vi "POM_PROM_ТЗЧ_host.vi"() -> ()   [LabVIEW 2013]
uses:
  <instrlib>/niDMM/nidmm.llb/niDMM Resolution in Digits.ctl
  <instrlib>/niDMM/nidmm.llb/niDMM Function.ctl
  <vilib>/Analysis/baseanly.llb/Mean (DBL).vi
  <instrlib>/niDMM/nidmm.llb/niDMM Configure Measurement Digits.vi
  <vilib>/Analysis/NI_AALBase.lvlib
  <instrlib>/niDCPower/nidcpower.llb/niDCPower Measurement Type.ctl
panel:
  in  "Нагрев":bool
  in  "В ручную":bool
  in  "Напряжение Пельтье":dbl=0.30000000000000004
  in  "milliseconds to wait 2":u32=75
  out "Monitor current, uA":dbl(graph)=0.07016814151938888
  in  "Порог типатиристора, мА":dbl=55.0
  out "Счетчик сбоев":dbl
  out "Температура":i32=25
  out "Образец":i32=2001
  out "Сеанс":i32
  out "Ион":string="Nope"
  in  "SEL simulation":bool
  out "refnum out":refnum<file>
  in  "Облучение!":bool
  out "Стабилизировано":bool
  in  "+ V TEC для новой точки":dbl=0.11 format="%#_13g"
  in  "Вычет для \"антиразгона\"":dbl format="%#_13g"
  in  "Оставить в раб.\nрежиме":bool
  out "Boolean":bool
  in  "Num_hits_req":u64=7
  out "Num_hits":u64
  in  "Count_hits?":bool
  in  "tstab между точками, мс":u32=1
  in  "Предел тока PDext, мА":dbl=20.0
  in  "Отладка(F)/\n/Рабочий(T)":bool=TRUE
  out "TEC_current, mA":dbl=27.478324133936702
  in  "Param_Log":path=path "D:/#rkm/FONONIWE-4/Logs_Dubna/POM"
  in  "trelax":u32=35000
  out "Volt_onRes":dbl=2.4602762193630356
  out "NoStab":bool
  out "Operating Current, mA":dbl=0.04490127125944435
  in  "Desirable Operating current, mA":dbl=50.0 format="%#_6f"
  out "Error message":string="Too much try"
  in  "Up_Volt_limit":dbl=5.0
  in  "Low_Volt_limit":dbl=1.0
  out "ThRes_stabil":bool=TRUE
  out "Подстроенное напряжение\nстабилизации":dbl=0.15911789062499992
  out "ThRes value":dbl=17926.2140625
  in  "Optimum ThRes":dbl=18000.0 format="%#_6f"
  in  "Предел тока LD, мА":dbl=100.0
  in  "Предел тока ТЕС, мА":dbl=300.0
  in  "Tab Control":enum32{"Page 1", "Page 2", "Page 3", "Page 4"}(tab)=enum."Page 4"
  out "RES(U_TEC) Graph":cluster{dbl[], dbl[]}(graph)={[-0.0, 0.025, 0.05, 0.07500000000000001, 0.1, 0.125, 0.15, 0.175, 0.19999999999999998, 0.22499999999999998, 0.24999999999999997, 0.27499999999999997, 0.3, 0.325, 0.35000000000000003, 0.37500000000000006, 0.4000000000000001, 0.4250000000000001, 0.4500000000000001, 0.47500000000000014, 0.5000000000000001, 0.5250000000000001, 0.5500000000000002, 0.5750000000000002, 0.6000000000000002, 0.6250000000000002, 0.6500000000000002, 0.6750000000000003, 0.7000000000000003, 0.7250000000000003, 0.7500000000000003, 0.7750000000000004], [15319.04365234375, 15328.19267578125, 15358.49169921875, 15409.562109375, 15479.3826171875, 15563.1861328125, 15668.50888671875, 15780.12734375, 15906.40224609375, 16043.244921875, 16186.97255859375, 16341.84609375, 16507.0697265625, 16676.522265625, 16856.963671875, 17044.884375, 17239.0294921875, 17436.3736328125, 17641.744140625, 17850.8728515625, 18071.7896484375, 18291.20625, 18518.965625, 18750.4271484375, 18987.4517578125, 19230.0744140625, 19480.026171875, 19731.8517578125, 19984.940234375, 20249.54140625, 20514.206640625, 20780.055078125]}
  out "RES(I_TEC) Graph":cluster{dbl[], dbl[]}(graph)={[0.03457500435386299, 4.049114950716204, 7.9212407853678135, 11.611043015146826, 15.078954849250364, 18.53827902856892, 21.88408259580828, 25.295266856430793, 28.546483256934756, 31.60504570629327, 34.77027313644012, 37.80993408960394, 40.856486299311584, 43.94949565069024, 47.03219408159836, 50.06845592920464, 52.92926046093485, 55.95350027659507, 58.865931959242474, 61.84202368829837, 64.7802788203752, 67.60156326899994, 70.44177990185035, 73.41963022613506, 76.46974363403558, 79.22741287887104, 82.2001312992484, 85.07135997639818, 88.0785044464861, 90.98931976346292, 93.95691599392462, 96.75420696595256], [15319.04365234375, 15328.19267578125, 15358.49169921875, 15409.562109375, 15479.3826171875, 15563.1861328125, 15668.50888671875, 15780.12734375, 15906.40224609375, 16043.244921875, 16186.97255859375, 16341.84609375, 16507.0697265625, 16676.522265625, 16856.963671875, 17044.884375, 17239.0294921875, 17436.3736328125, 17641.744140625, 17850.8728515625, 18071.7896484375, 18291.20625, 18518.965625, 18750.4271484375, 18987.4517578125, 19230.0744140625, 19480.026171875, 19731.8517578125, 19984.940234375, 20249.54140625, 20514.206640625, 20780.055078125]}
  out "I_PD_Ext(I_LD) Graph":cluster{dbl[], dbl[]}(graph)={[0.0, 5.125820672560687, 10.202363077068034, 15.09070291650038, 20.026524721844005, 24.848748653112324, 29.706585438813228, 34.55255888002156, 39.41379829521783, 44.31743313126964, 49.35841653002704], [0.6213749657825949, 0.6126206411732633, 0.5986137214569519, 0.5846068013204628, 0.5933611264550083, 0.5670981505590477, 0.5355825775341941, 0.586357666360488, 0.5355825775341941, 0.5478386339632713, 0.5390843079753067]}
  out "I_PD(I_LD) Graph":cluster{dbl[], dbl[]}(graph)={[0.0, 5.125820672560687, 10.202363077068034, 15.09070291650038, 20.026524721844005, 24.848748653112324, 29.706585438813228, 34.55255888002156, 39.41379829521783, 44.31743313126964, 49.35841653002704], [0.00446055423708458, 0.1890051237296575, 1.3185992656872259, 47.69851657329127, 96.3842059718445, 145.3466946259141, 195.95923949964345, 243.1108383461833, 288.08951028622687, 334.6654470078647, 377.8655605856329]}
  out "I_pd, uA":dbl
  out "IPD(ext), mA":dbl
  out "V2(I_LD) Graph":cluster{dbl[], dbl[]}(graph)={[0.0, 5.125820672560687, 10.202363077068034, 15.09070291650038, 20.026524721844005, 24.848748653112324, 29.706585438813228, 34.55255888002156, 39.41379829521783, 44.31743313126964, 49.35841653002704], [0.0006418486043783589, 1.1699665507043246, 1.452329111789965, 1.6798119558569469, 1.9201177244634586, 2.150803801269446, 2.3862573437846697, 2.612869753183121, 2.8439823589319366, 3.0683008415602466, 3.3013683877429134]}
  out "Forward Voltage, V":dbl
  out "OP(I_LD) Graph":cluster{dbl[], dbl[]}(graph)={[0.0, 5.125820672560687, 10.202363077068034, 15.09070291650038, 20.026524721844005, 24.848748653112324, 29.706585438813228, 34.55255888002156, 39.41379829521783, 44.31743313126964, 49.35841653002704], [0.0, 0.0, 0.02, 0.74, 1.5, 2.27, 3.0300000000000002, 3.8, 4.58, 5.33, 6.119999999999999]}
  out "Ophir, mW":dbl
  out "Пороговый ток":dbl
  out "ExtPhotodiode Current":dbl(graph)
  out "Boolean 2":bool
  out "Сопротивление терморез-ра":dbl(graph)=16035.80078125
  out "thRes_adj":dbl=16035.80078125 format="%0.2f"
  in  "Source-Ohm w8":u32=1000
  in  "Coeff_High":dbl=90000.0 format="%#_13g"
  in  "Coeff_low":dbl=20000.0 format="%#_13g"
  in  "Coeff_thr":dbl=1500.0
  out "+Voltage\nrequired":dbl=0.0008410915798611111
  out "Разница ThRes":dbl=75.6982421875
  out "Operating Current":dbl(graph)
  out "Готовы облучать":bool
  out "accommodated voltage (out)":dbl=5.701287315779691
  in  "4070_Rele_source":enum16{"S2_Ch0", "S1_Ch2"}(ring)
  in  "the upper limit for the voltage_LD":dbl=6.0
  in  "the lower limit for the voltage_LD":dbl=1.0
  in  "Start voltage_LD":dbl=2.0 format="%#.7f"
  in  "accuracy_LD":dbl=0.01 step=0.01
  in  "Res_LD":dbl=50.0
  in  "TEC_Source":enum16{"S1_Ch2", "S2_Ch0", "S3_Ch1"}(ring)
  in  "Start voltage":dbl=0.1 format="%#.7f"
  in  "the upper limit for the voltage":dbl=0.8
  in  "the lower limit for the voltage":dbl
  in  "Точность ThRes":dbl=75.0 step=0.01
  out "Ro, Ом":dbl=15321.56484375
  in  "OphirLMMeasurementLib.ICoLMMeasurement":refnum<k7>
  out "hDevice":i32=1004
  out "Ophir_address":refnum<k7>
  in  "Power Enable":bool
  in  "4071(2)":refnum<k15>="PXI1Slot4_2"
  out "4071(2)_adress":refnum<k15>="PXI1Slot4_2 (12)" caption="4071(1)_out"
  in  "4071(1)":refnum<k15>="Dev5"
  out "4071(1)_adress":refnum<k15>="Dev5 (5)" caption="4071(1)_out"
  out "4070_address":refnum<k15>="PXI4Slot10 (5)" caption="4070_out"
  in  "4070":refnum<k15>="PXI4Slot10"
  in  "Source_3":refnum<k15>
  out "Source_3_Vcc_out":refnum<k15> caption="S_3_out"
  out "Source_2_Vcc_out":refnum<k15>="PXI4Slot2" caption="S_2_out"
  in  "Source_2":refnum<k15>="PXI4Slot2"
  out "Source_1_Vcc_out":refnum<k15>="PXI4Slot4" caption="S_1_out"
  in  "Source_1":refnum<k15>="PXI4Slot4"
  out "Прервать":bool=TRUE
  in  "milliseconds to wait":u32=2000
  in  "Шаг напр\nдля TEC, В":dbl=0.025
  in  "Начальное\nнапряжение TEC, В":dbl
  in  "кол-во точек для TEC":i32=32
  in  "stop":bool
  in  "Case":T1(ring)=enum."Quit"
  out "Выполняется":bool
  in  "Раб. режим LD":bool
  in  "Хар-ка TEC":bool
  in  "Хар-ки от I_LD":bool
  out "Status:":string="IDLE"
  out "Подстроенный ток, mA":dbl=50.042267338193476
  in  "Шаг, мА":dbl=5.0
  in  "Начальный ток, мА":dbl
  in  "Кол-во точек":i32=11
  # "20"
  # "7"
  # "5"
  # "ток Пельтье во время стабилизации"
  # "0,15"
  # "Охлаждение"
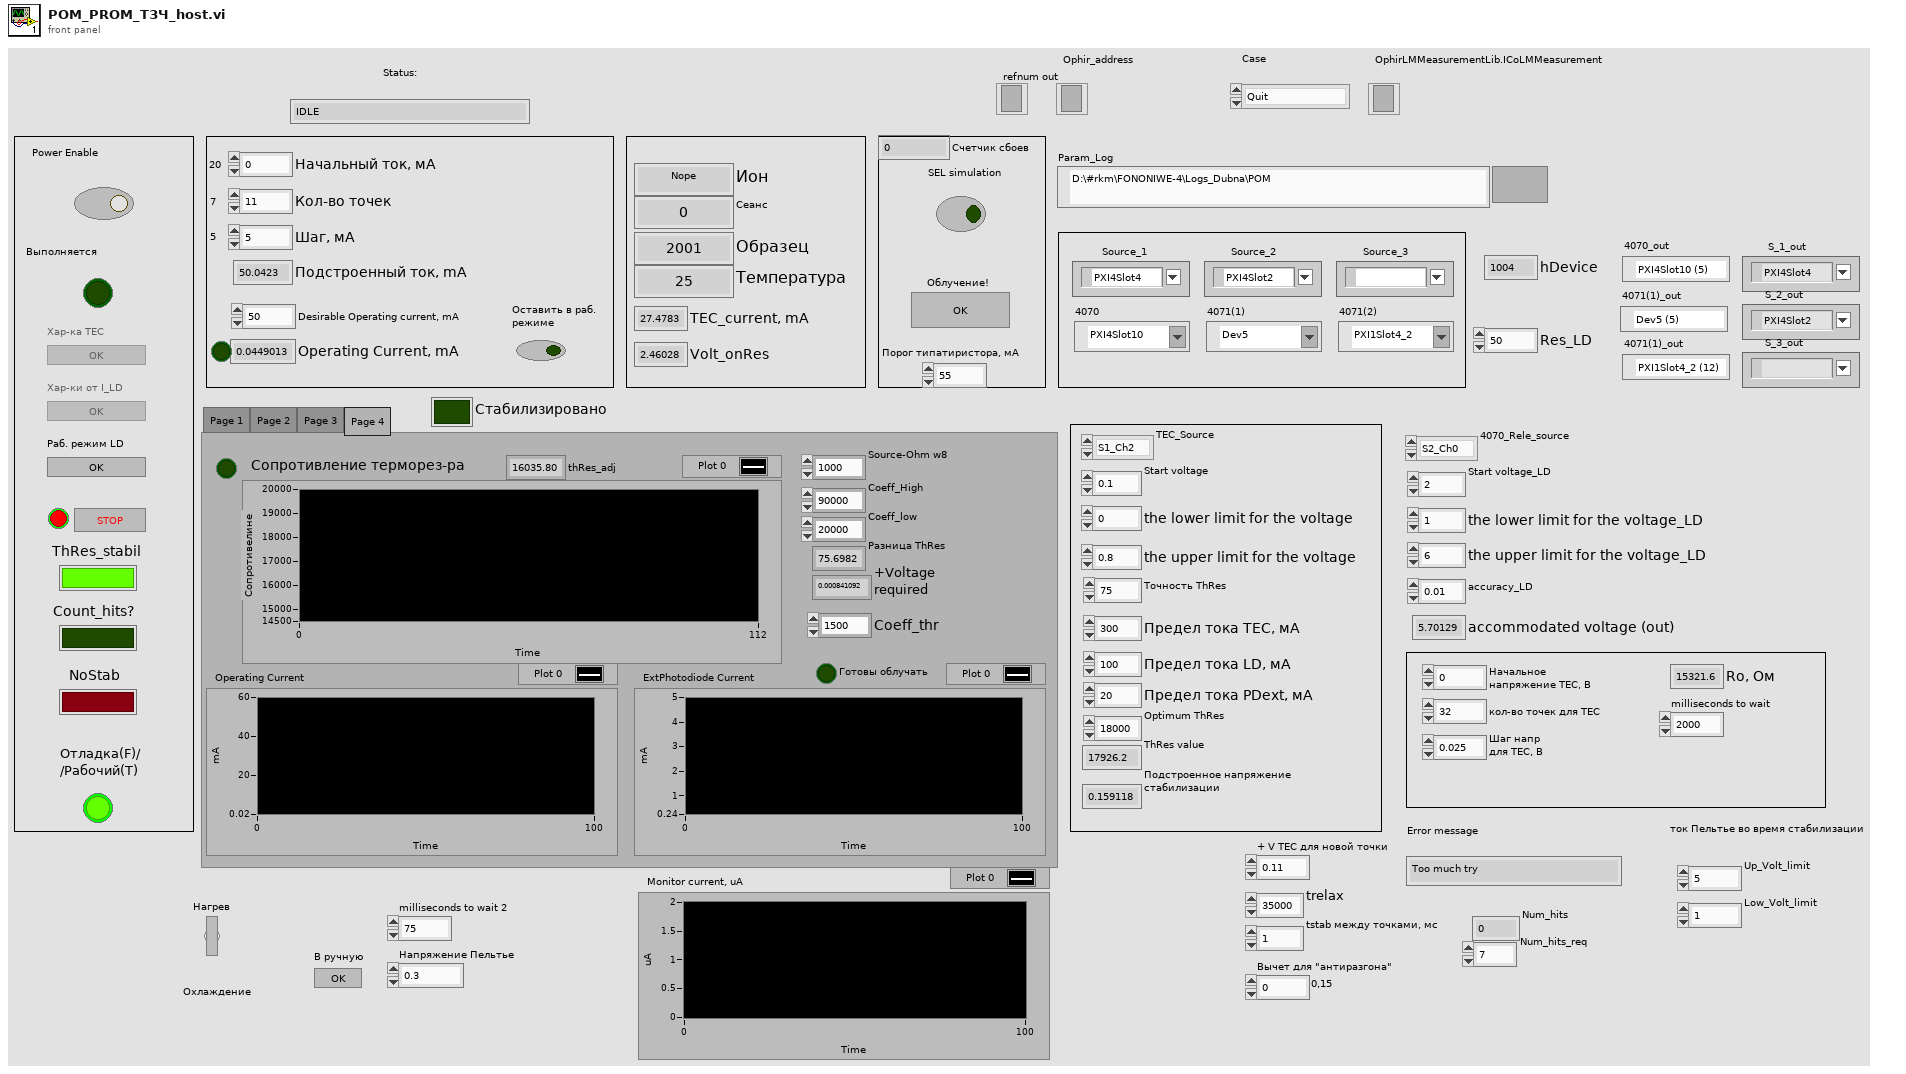
[diagram p1: front panel]
types:
  T1 = enum16{"Initialization", "TEC_Chars", "TRes_Check(Idle)", "Characteristics", "Bias", "Quit"}
  T2 = typedef "niDMM Function.ctl" = enum16{"DC Volts", "AC Volts", "DC Current", "AC Current", "2-wire Resistance", "4-wire Resistance", "Diode", "Frequency", "Period", "AC Volts DC Coupled", "Capacitance", "Inductance", "Temperature"}
  T3 = enum8{"Enabled", "Disabled", "Disabled and Grayed Out"}
  T4 = typedef "niDMM Resolution in Digits.ctl" = dbl
  T5 = enum16{"open", "replace", "create", "open or create", "replace or create", "replace or create with confirmation"}
  T6 = typedef "niDCPower Measurement Type.ctl" = i32
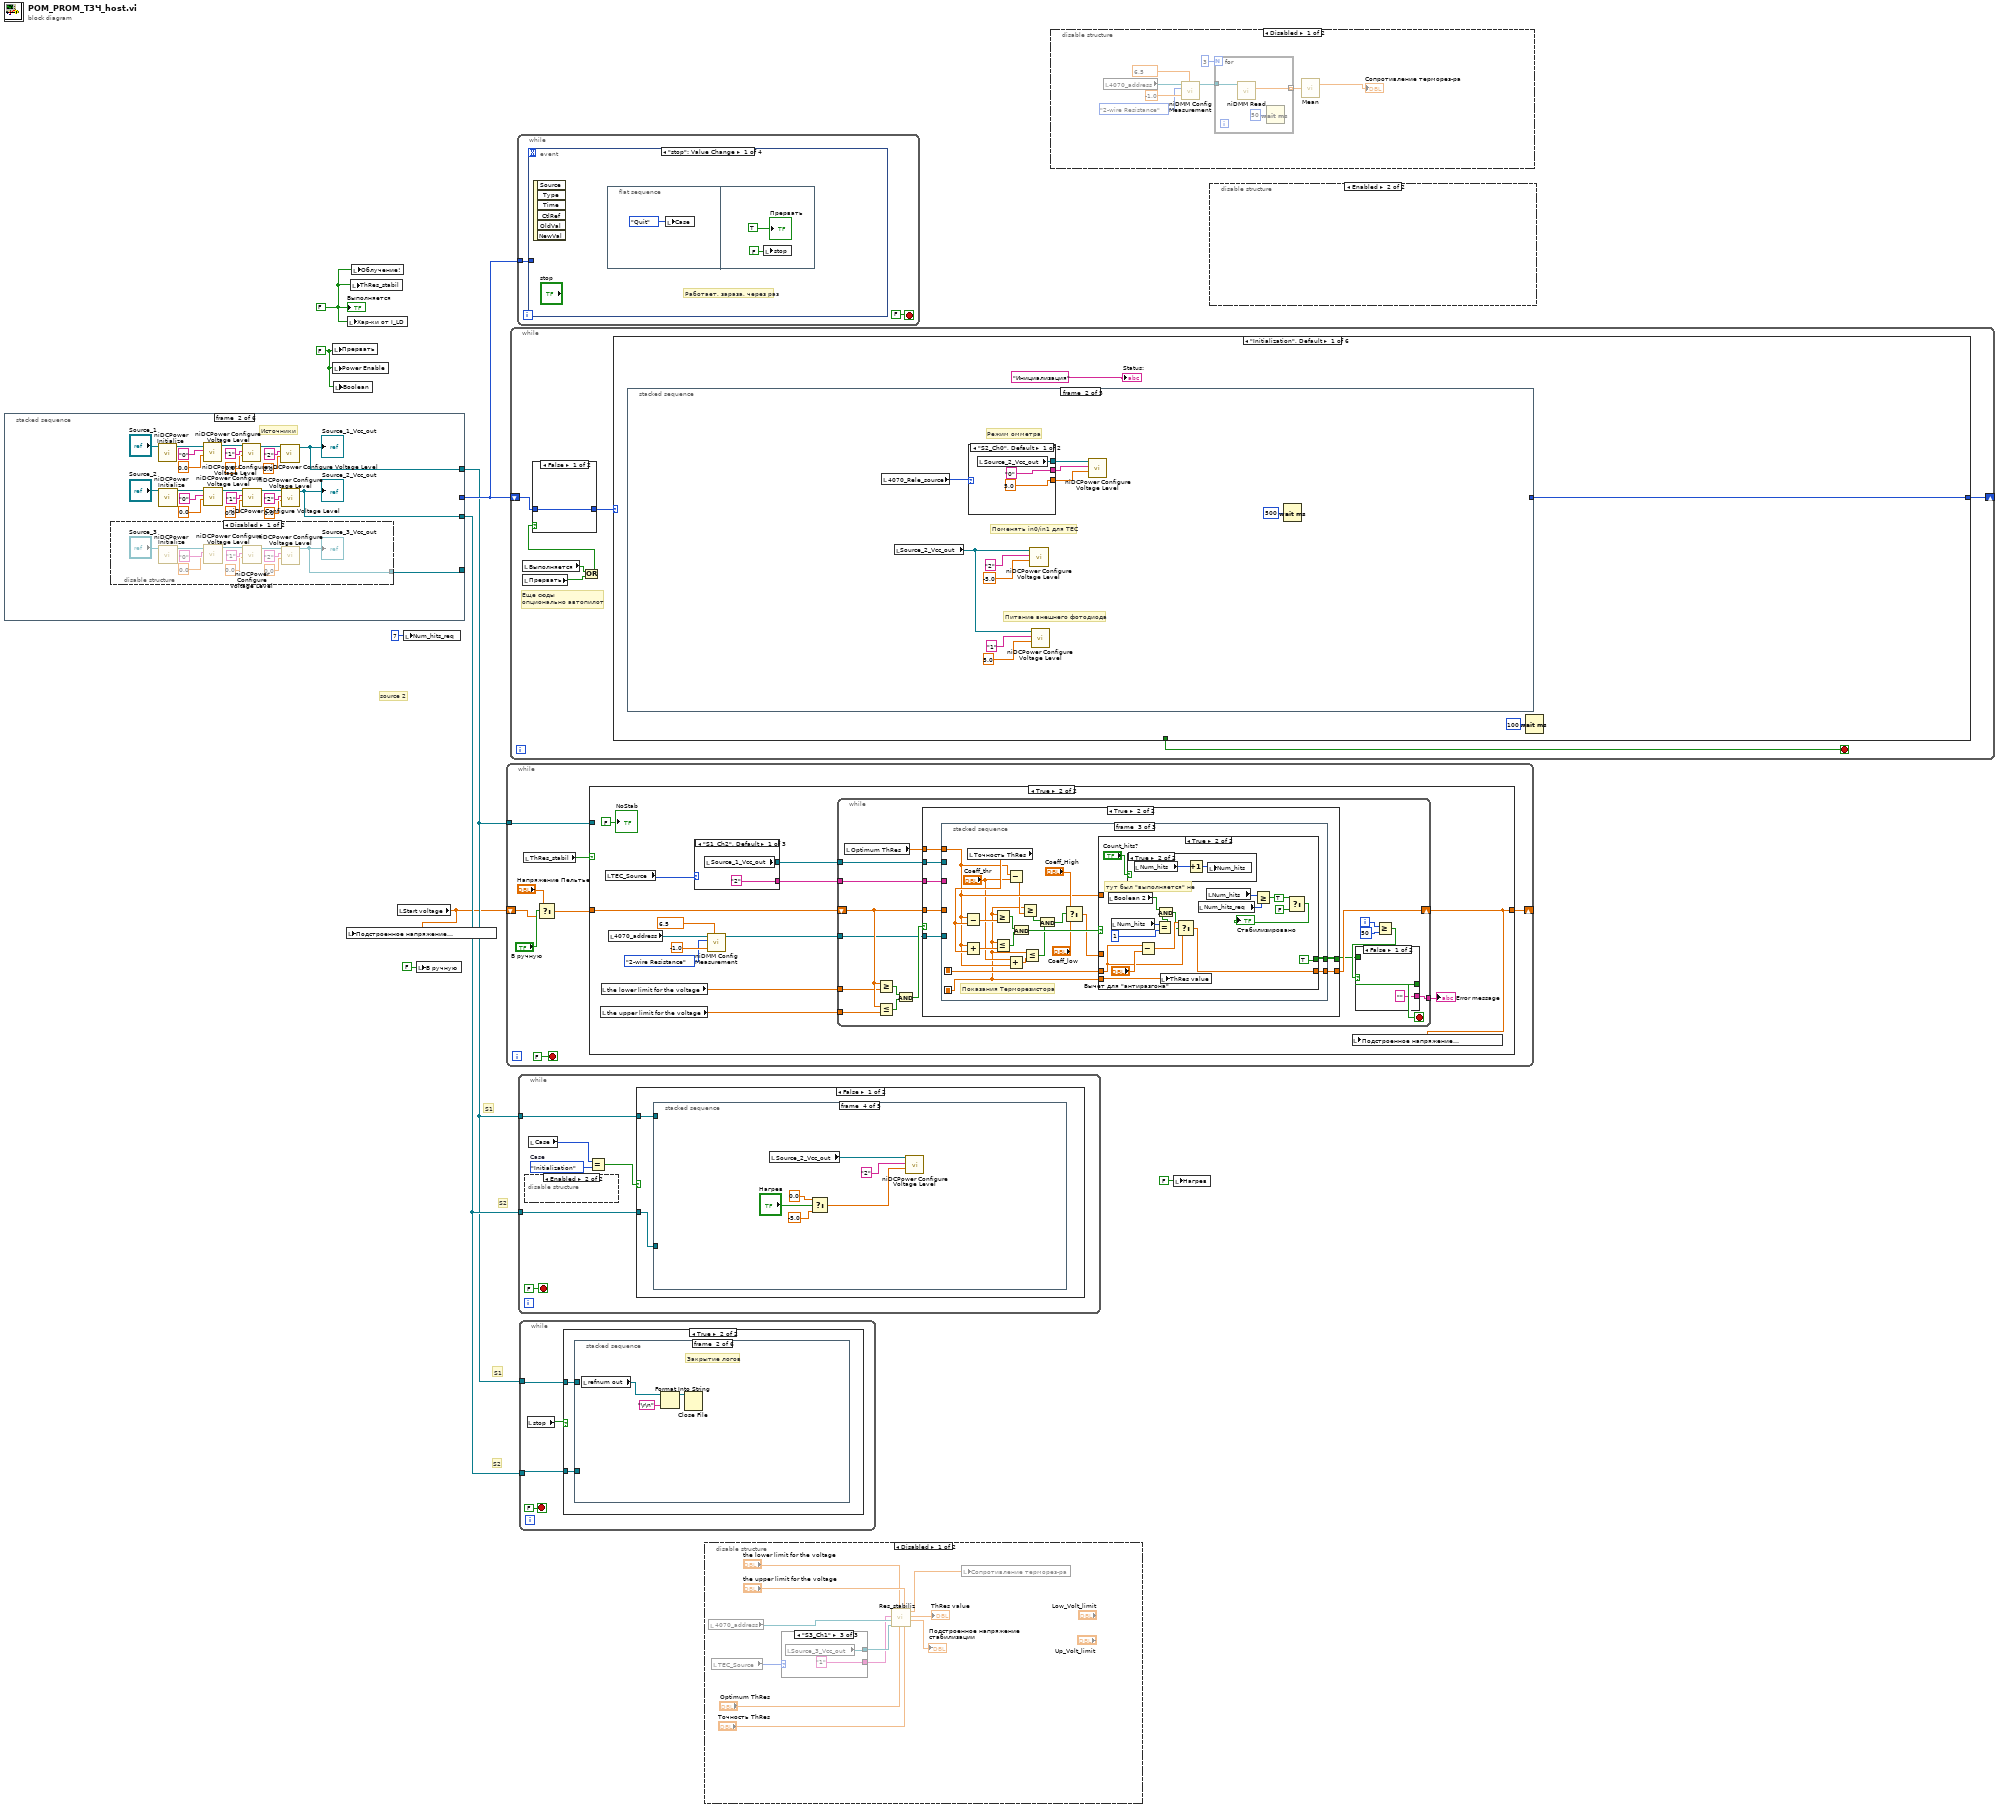
[diagram p0: block diagram]
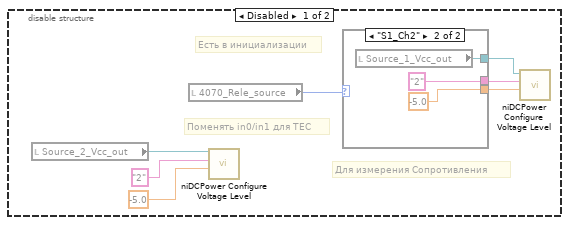
[diagram p3: hidden frame]
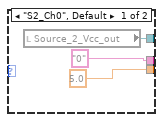
[diagram p4: hidden frame]
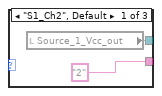
[diagram p5: hidden frame]
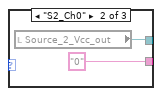
[diagram p6: hidden frame]
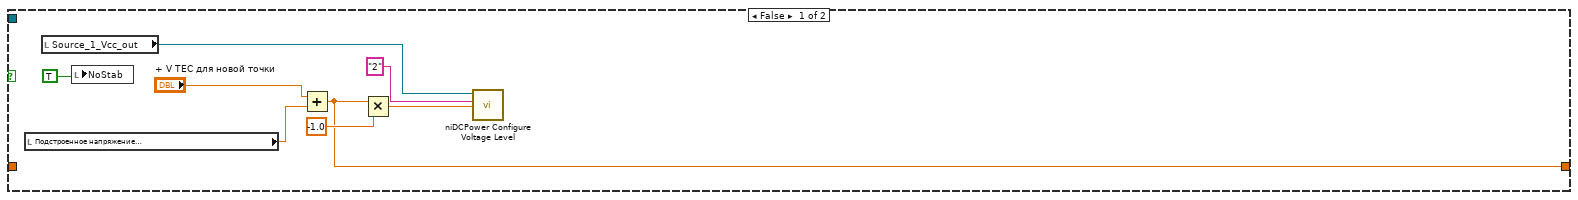
[diagram p8: hidden frame]
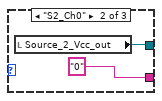
[diagram p9: hidden frame]
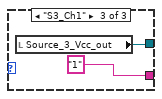
[diagram p10: hidden frame]
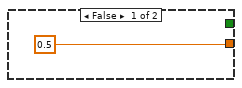
[diagram p11: hidden frame]
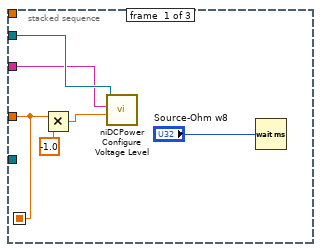
[diagram p12: hidden frame]
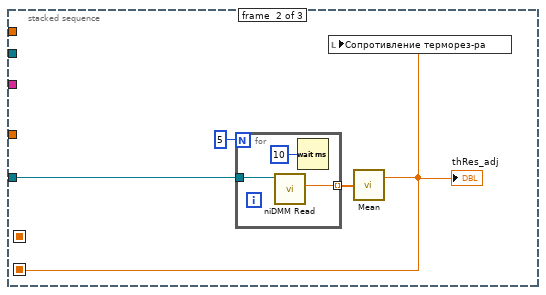
[diagram p13: hidden frame]
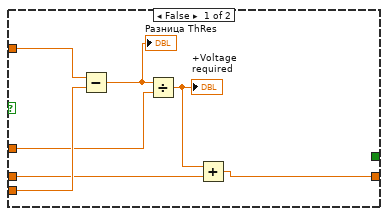
[diagram p14: hidden frame]
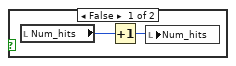
[diagram p15: hidden frame]
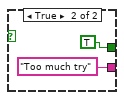
[diagram p16: hidden frame]
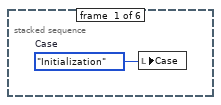
[diagram p18: hidden frame]
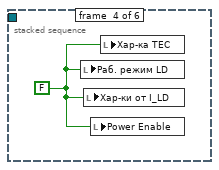
[diagram p20: hidden frame]
diagram:
  w4 = FALSE
  w6 = FALSE
  # "source 2"
  # "S1"
  # "S2"
  # "S2"
  # "S1"
  n1 = stacked-sequence {
    tunnel: [_ _ _ _ _ w93] -> w9
    tunnel: [_ w20 _ _ _ _] -> w8
    tunnel: [_ w19 _ _ _ _] -> w7
    tunnel: [_ w18 _ _ _ _] -> _
    frame #0 {
      n2 = while {
        stop <- w16 stop-if-true
        w11 = T3."Disabled and Grayed Out" ("Disabled")
        n3 = local write "Стабилизировано"(FALSE) -> ()
        n4 = property on="Хар-ка TEC" class="Bool (strict)"("DisabledEnum"=w11) -> ()  [unwired: 2 in, 2 out]
        n5 = property on="Раб. режим LD" class="Bool (strict)"("DisabledEnum"=w11) -> ()  [unwired: 2 in, 2 out]
        n6 = property on="Хар-ки от I_LD" class="Bool (strict)"("DisabledEnum"=w11) -> ()  [unwired: 2 in, 2 out]
        n7 = local write "Status:"("Ожидание Power Enable" ("Status:")) -> ()
        n8 = local read "stop"() -> (w14:bool)
        n9 = case shown="True" w14 {
          frame False {
          }
          frame True {
            n10 = local write "Прервать"(TRUE) -> ()
          }
        }
        n11 = Or(x=w14, y="Power Enable") -> (x .or. y?=w16:bool)
        n12 = Wait (ms)(milliseconds to wait=u32 100) -> ()  [unwired: 1 out]
      }
    }
    frame #1 {
      # "Источники"
      n13 = disable-structure shown="Disabled" {
        disable-tunnel: [w41 _] -> w18
        frame Disabled {
          n14 = call <instrlib>:"niDCPower Initialize.vi"("resource name"="Source_3") -> ("instrument handle out"=w45:refnum<k15>)  [unwired: 3 in, 7 out]
          n15 = call <instrlib>:"niDCPower Configure Voltage Level.vi"("voltage level"=0.0, "channel name"="0", "instrument handle"=w45) -> ("instrument handle out"=w44:refnum<k15>)  [unwired: 7 in, 1 out]
          n16 = call <instrlib>:"niDCPower Configure Voltage Level.vi"("voltage level"=0.0, "channel name"="1", "instrument handle"=w44) -> ("instrument handle out"=w50:refnum<k15>)  [unwired: 7 in, 1 out]
          n17 = call <instrlib>:"niDCPower Configure Voltage Level.vi"("voltage level"=0.0, "channel name"="2", "instrument handle"=w50) -> ("instrument handle out"=w41:refnum<k15>)  [unwired: 7 in, 1 out]
          "Source_3_Vcc_out" <- w41
        }
        frame Enabled {
        }
      }
      n18 = call <instrlib>:"niDCPower Initialize.vi"("resource name"="Source_1") -> ("instrument handle out"=w34:refnum<k15>)  [unwired: 3 in, 7 out]
      n19 = call <instrlib>:"niDCPower Initialize.vi"("resource name"="Source_2") -> ("instrument handle out"=w27:refnum<k15>)  [unwired: 3 in, 7 out]
      n20 = call <instrlib>:"niDCPower Configure Voltage Level.vi"("voltage level"=0.0, "channel name"="0", "instrument handle"=w34) -> ("instrument handle out"=w33:refnum<k15>)  [unwired: 7 in, 1 out]
      n21 = call <instrlib>:"niDCPower Configure Voltage Level.vi"("voltage level"=0.0, "channel name"="0", "instrument handle"=w27) -> ("instrument handle out"=w28:refnum<k15>)  [unwired: 7 in, 1 out]
      n22 = call <instrlib>:"niDCPower Configure Voltage Level.vi"("voltage level"=0.0, "channel name"="1", "instrument handle"=w33) -> ("instrument handle out"=w40:refnum<k15>)  [unwired: 7 in, 1 out]
      n23 = call <instrlib>:"niDCPower Configure Voltage Level.vi"("voltage level"=0.0, "channel name"="1", "instrument handle"=w28) -> ("instrument handle out"=w22:refnum<k15>)  [unwired: 7 in, 1 out]
      n24 = call <instrlib>:"niDCPower Configure Voltage Level.vi"("voltage level"=0.0, "channel name"="2", "instrument handle"=w40) -> ("instrument handle out"=w19:refnum<k15>)  [unwired: 7 in, 1 out]
      "Source_1_Vcc_out" <- w19
      n25 = call <instrlib>:"niDCPower Configure Voltage Level.vi"("voltage level"=0.0, "channel name"="2", "instrument handle"=w22) -> ("instrument handle out"=w20:refnum<k15>)  [unwired: 7 in, 1 out]
      "Source_2_Vcc_out" <- w20
    }
    frame #2 {
      w52 = T4 6.5 items=["3 1/2"=3.5, "4 1/2"=4.5, "5 1/2"=5.5, "6 1/2"=6.5, "7 1/2"=7.5] ("Resolution in Digits")
      w54 = TRUE ("Reset")
      (unwired) enum16{"S1_Ch2", "S2_Ch0", "S3_Ch1"}."S1_Ch2"  # TEC_Source
      w65 = T4 6.5 items=["3 1/2"=3.5, "4 1/2"=4.5, "5 1/2"=5.5, "6 1/2"=6.5, "7 1/2"=7.5] ("Resolution in Digits")
      w63 = TRUE ("Reset")
      # "4065"
      # "4070"
      # "Мультиметры"
      n26 = disable-structure shown="Disabled" {
        frame Disabled {
          w72 = T4 7.5 items=["3 1/2"=3.5, "4 1/2"=4.5, "5 1/2"=5.5, "6 1/2"=6.5, "7 1/2"=7.5] ("Resolution in Digits")
          w70 = TRUE ("Reset")
          # "4071"
          n27 = call <instrlib>:"niDMM Initialize.vi"("Reset"=w70, "ID Query"=w70, "Instrument Descriptor"="4071(2)") -> ("instrument handle out"=w68:refnum<k15>)  [unwired: 7 in, 1 out]
          n28 = call-poly <instrlib>:"niDMM Config Measurement.vi"("Range"=-1.0 ("Configuration:Measurement Options:Max Frequency"), "Resolution in Digits"=w72, "Function"=niDMM_Function."DC Current" ("multimeter mode"), "instrument handle"=w68) -> ("instrument handle out"=w66:refnum<k15>)  [unwired: 6 in, 1 out]
          "4071(2)_adress" <- w66
          n29 = call <instrlib>:"niDMM Read.vi"("instrument handle"=w66) -> ()  [unwired: 8 in, 3 out]
        }
        frame Enabled {
        }
      }
      n30 = call <instrlib>:"niDMM Initialize.vi"("Reset"=w54, "ID Query"=w54, "Instrument Descriptor"="4071(1)") -> ("instrument handle out"=w56:refnum<k15>)  [unwired: 7 in, 1 out]
      n31 = call <instrlib>:"niDMM Initialize.vi"("Reset"=w63, "ID Query"=w63, "Instrument Descriptor"="4070") -> ("instrument handle out"=w61:refnum<k15>)  [unwired: 7 in, 1 out]
      n32 = call-poly <instrlib>:"niDMM Config Measurement.vi"("Range"=-1.0 ("Configuration:Measurement Options:Max Frequency"), "Resolution in Digits"=w52, "Function"=niDMM_Function."DC Current" ("multimeter mode"), "instrument handle"=w56) -> ("instrument handle out"=w58:refnum<k15>)  [unwired: 6 in, 1 out]
      "4071(1)_adress" <- w58
      n33 = call-poly <instrlib>:"niDMM Config Measurement.vi"("Range"=-1.0 ("Configuration:Measurement Options:Max Frequency"), "Resolution in Digits"=w65, "Function"=niDMM_Function."DC Current" ("multimeter mode"), "instrument handle"=w61) -> ("instrument handle out"=w59:refnum<k15>)  [unwired: 6 in, 1 out]
      "4070_address" <- w59
      n34 = call <instrlib>:"niDMM Read.vi"("instrument handle"=w58) -> ()  [unwired: 8 in, 3 out]
      n35 = call <instrlib>:"niDMM Read.vi"("instrument handle"=w59) -> ()  [unwired: 8 in, 3 out]
    }
    frame #3 {
      n36 = disable-structure shown="Disabled" {
        frame Disabled {
          n37 = Automation Open(Automation Refnum="OphirLMMeasurementLib.ICoLMMeasurement") -> (Automation Refnum=w81:refnum<k7>)  [unwired: 3 in, 1 out]
          n38 = invoke class="ICoLMMeasurement" method="ScanUSB"(reference=w81) -> (reference out=w83:refnum<k7>, "serialNumbers"=w80:variant)  [unwired: 3 in, 2 out]
          "Ophir_address" <- w83
          n39 = Variant To Data(type=string[] [], Variant=w80) -> (data=w79:string[])  [unwired: 1 in, 1 out]
          n40 = Index Array(array=w79, index=0) -> (element=w76:string)
          n41 = invoke class="ICoLMMeasurement" method="OpenUSBDevice"(reference=w83, "serialNumber"=w76) -> (reference out=w75:refnum<k7>, "hDevice"=w74:i32)  [unwired: 3 in, 3 out]
          "hDevice" <- w74
          n42 = invoke class="ICoLMMeasurement" method="StartStream"(reference=w75, "hDevice"=w74, "channel"=0) -> ()  [unwired: 2 in, 5 out]
        }
        frame Enabled {
        }
      }
    }
    frame #4 {
      n43 = while {
        stop <- w85 stop-if-true
        n44 = call "Save_dialogue_number_ION.vi"() -> ("Температура 2"=→"Температура":i32, "Номер образца 2"=→"Образец":i32, "Номер сеанса 2"=→"Сеанс":i32, "Ион 2"=→"Ион":string, "OK Button 2"=w85:bool)  [unwired: 5 in]
        n45 = Wait (ms)(milliseconds to wait=u32 250) -> ()  [unwired: 1 out]
      }
      "Счетчик сбоев" <- 0.0
    }
    frame #5 {
      (unwired) enum16{"S2_Ch0", "S1_Ch2"}."S2_Ch0"  # 4070_Rele_source
      w93 = T1."Initialization"  # Case
      n46 = property on="Сопротивление терморез-ра" class="WFChart (strict)"("History Data"=dbl[] []) -> ()  [unwired: 2 in, 2 out]
      n47 = local write "Start voltage"("Start voltage") -> ()
    }
  }
  n48 = local write "Прервать"(w6) -> ()
  n49 = local write "Power Enable"(w6) -> ()
  n50 = local write "Boolean"(w6) -> ()
  n51 = local write "Хар-ки от I_LD"(w4) -> ()
  n52 = local write "ThRes_stabil"(w4) -> ()
  n53 = local write "Облучение!"(w4) -> ()
  n54 = local read "Start voltage"() -> (w5:dbl)
  n55 = local write "Подстроенное напряжение\nстабилизации"(w5) -> ()
  n56 = local write "Num_hits_req"(u64 7 ("Num_hits_req")) -> ()
  n57 = local write "В ручную"(FALSE ("В ручную")) -> ()
  n58 = while {
    shift-right: [w99] -> _
    shift-left: w5 -> [w95]
    tunnel: w7 -> [w98]
    stop <- FALSE stop-if-true
    n59 = local read "ThRes_stabil"() -> (w100:bool)
    n60 = Select(t="Напряжение Пельтье", s="В ручную", f=w95) -> (s? t:f=w94:dbl)
    n61 = case shown="True" w100 {
      tunnel: [w103 w111] -> w99
      tunnel: w94 -> [_ w117]
      tunnel: w98 -> [_ _]
      frame False {
        n62 = local read "Подстроенное напряжение\nстабилизации"() -> (w102:dbl)
        n63 = local read "Source_1_Vcc_out"() -> (w107:refnum<k15>)
        n64 = local write "NoStab"(TRUE) -> ()
        n65 = Add(x="+ V TEC для новой точки", y=w102) -> (x+y=w103:dbl)
        n66 = Multiply(x=w103, y=-1.0) -> (x*y=w104:dbl)
        n67 = call <instrlib>:"niDCPower Configure Voltage Level.vi"("voltage level"=w104, "channel name"="2", "instrument handle"=w107) -> ()  [unwired: 7 in, 2 out]
      }
      frame True {
        w113 = T4 6.5 items=["3 1/2"=3.5, "4 1/2"=4.5, "5 1/2"=5.5, "6 1/2"=6.5, "7 1/2"=7.5] ("Resolution in Digits")
        n68 = local read "the upper limit for the voltage"() -> (w118:dbl)
        n69 = local read "the lower limit for the voltage"() -> (w119:dbl)
        n70 = local read "TEC_Source"() -> (w120:enum16{"S1_Ch2", "S2_Ch0", "S3_Ch1"})
        n71 = local read "4070_address"() -> (w112:refnum<k15>)
        n72 = case shown="\"S1_Ch2\", Default" w120 {
          tunnel: [w125 w127 w129] -> w122
          tunnel: ["2" "0" "1"] -> w121
          frame "S1_Ch2", Default {
            n73 = local read "Source_1_Vcc_out"() -> (w125:refnum<k15>)
          }
          frame "S2_Ch0" {
            n74 = local read "Source_2_Vcc_out"() -> (w127:refnum<k15>)
          }
          frame "S3_Ch1" {
            n75 = local read "Source_3_Vcc_out"() -> (w129:refnum<k15>)
          }
        }
        n76 = call-poly <instrlib>:"niDMM Config Measurement.vi"("Range"=-1.0 ("Configuration:Measurement Options:Max Frequency"), "Resolution in Digits"=w113, "Function"=niDMM_Function."2-wire Resistance" ("multimeter mode"), "instrument handle"=w112) -> ("instrument handle out"=w110:refnum<k15>)  [unwired: 6 in, 1 out]
        n77 = while {
          tunnel: w121 -> [w137]
          tunnel: w122 -> [w138]
          tunnel: w110 -> [w136]
          shift-right: [w135] -> w111
          shift-left: w117 -> [w139]
          tunnel: [w133] -> w123
          tunnel: w119 -> [w131]
          tunnel: w118 -> [w130]
          i -> [w143]
          stop <- w144 stop-if-true
          n78 = local read "Optimum ThRes"() -> (w132:dbl)
          n79 = Greater Or Equal?(x=w139, y=w131) -> (x >= y?=w142:bool)
          n80 = Less Or Equal?(x=w139, y=w130) -> (x <= y?=w141:bool)
          n81 = And(x=w142, y=w141) -> (x .and. y?=w140:bool)
          n82 = case shown="True" w140 {
            tunnel: w139 -> [_ w152]
            tunnel: w138 -> [_ w154]
            tunnel: w137 -> [_ w153]
            tunnel: w132 -> [_ w150]
            tunnel: w136 -> [_ w151]
            tunnel: [0.5 w149] -> w135
            tunnel: [_ w148] -> w134
            frame False {
            }
            frame True {
              n83 = stacked-sequence {
                seq-local: [w155 _ _] -> [_ _ w182]
                seq-local: [_ w162 _] -> [_ _ w172]
                tunnel: w154 -> [w160 _ _]
                tunnel: w153 -> [w159 _ _]
                tunnel: w152 -> [w155 _ _]
                tunnel: w151 -> [_ w161 _]
                tunnel: w150 -> [_ _ w175]
                tunnel: [_ _ w181] -> w149
                tunnel: [_ _ w180] -> w148
                frame #0 {
                  n84 = Multiply(x=w155, y=-1.0) -> (x*y=w156:dbl)
                  n85 = call <instrlib>:"niDCPower Configure Voltage Level.vi"("voltage level"=w156, "channel name"=w159, "instrument handle"=w160) -> ()  [unwired: 7 in, 2 out]
                  n86 = Wait (ms)(milliseconds to wait="Source-Ohm w8") -> ()  [unwired: 1 out]
                }
                frame #1 {
                  n87 = for {
                    N: 5 -> [_]
                    tunnel: w161 -> [w167]
                    tunnel: [w166] -> w163 mode=indexing
                    n88 = call <instrlib>:"niDMM Read.vi"("instrument handle"=w167) -> ("Measurement"=w166:dbl)  [unwired: 8 in, 2 out]
                    n89 = Wait (ms)(milliseconds to wait=u32 10) -> ()  [unwired: 1 out]
                  }
                  n90 = call-poly <vilib>:"Mean.vi"("X"=w163) -> ("mean"=w162:dbl)  [unwired: 1 out]
                  "thRes_adj" <- w162
                  n91 = local write "Сопротивление терморез-ра"(w162) -> ()
                }
                frame #2 {
                  # "Показания Терморезистора"
                  n92 = local read "Точность ThRes"() -> (w179:dbl)
                  n93 = Subtract(x=w175, y=w179) -> (x-y=w185:dbl)
                  n94 = Add(x=w175, y=w179) -> (x+y=w186:dbl)
                  n95 = Greater Or Equal?(x=w172, y=w185) -> (x >= y?=w187:bool)
                  n96 = Less Or Equal?(x=w172, y=w186) -> (x <= y?=w184:bool)
                  n97 = Subtract(x=w175, y="Coeff_thr") -> (x-y=w173:dbl)
                  n98 = Add(x="Coeff_thr", y=w175) -> (x+y=w171:dbl)
                  n99 = And(x=w187, y=w184) -> (x .and. y?=w183:bool)
                  n100 = Greater Or Equal?(x=w172, y=w173) -> (x >= y?=w170:bool)
                  n101 = Less Or Equal?(x=w172, y=w171) -> (x <= y?=w169:bool)
                  n102 = And(x=w170, y=w169) -> (x .and. y?=w168:bool)
                  n103 = Select(t="Coeff_High", s=w168, f="Coeff_low") -> (s? t:f=w176:dbl)
                  n104 = case shown="True" w183 {
                    tunnel: [w189 w204] -> w181
                    tunnel: w182 -> [w191 w205]
                    tunnel: [_ TRUE] -> w180
                    tunnel: w172 -> [w192 w211]
                    tunnel: w175 -> [w193 _]
                    tunnel: w176 -> [w188 _]
                    frame False {
                      n105 = Subtract(x=w193, y=w192) -> (x-y=w194:dbl)
                      "Разница ThRes" <- w194
                      n106 = Divide(x=w194, y=w188) -> (x/y=w190:dbl)
                      "+Voltage\nrequired" <- w190
                      n107 = Add(x=w190, y=w191) -> (x+y=w189:dbl)
                    }
                    frame True {
                      # "тут был \"выполняется\" не"
                      n108 = local read "Boolean 2"() -> (w195:bool)
                      n109 = local read "Num_hits"() -> (w209:u64)
                      n110 = case shown="True" "Count_hits?" {
                        frame False {
                          n111 = local read "Num_hits"() -> (w213:u64)
                          n112 = Increment(x=w213) -> (x+1=w214:u64)
                          n113 = local write "Num_hits"(w214) -> ()
                        }
                        frame True {
                          n114 = local read "Num_hits"() -> (w216:u64)
                          n115 = Increment(x=w216) -> (x+1=w215:u64)
                          n116 = local write "Num_hits"(w215) -> ()
                        }
                      }
                      n117 = Subtract(x=w205, y="Вычет для \"антиразгона\"") -> (x-y=w206:dbl)
                      n118 = Equal?(x=w209, y=1) -> (x = y?=w203:bool)
                      n119 = And(x=w195, y=w203) -> (x .and. y?=w202:bool)
                      n120 = local write "ThRes value"(w211) -> ()
                      n121 = Select(t=w206, s=w202, f=w205) -> (s? t:f=w204:dbl)
                      n122 = local read "Num_hits_req"() -> (w200:u64)
                      n123 = local read "Num_hits"() -> (w201:u64)
                      n124 = Greater Or Equal?(x=w201, y=w200) -> (x >= y?=w199:bool)
                      n125 = Select(t=TRUE, s=w199, f=FALSE) -> (s? t:f=→"Стабилизировано":bool)
                    }
                  }
                }
              }
            }
          }
          n126 = Greater Or Equal?(x=w143, y=50) -> (x >= y?=w145:bool)
          n127 = case shown="False" w145 {
            tunnel: ["" "Too much try"] -> w133
            tunnel: [w218 TRUE] -> w144
            tunnel: w134 -> [w218 _]
            frame False {
            }
            frame True {
            }
          }
        }
        "Error message" <- w123
        n128 = local write "Подстроенное напряжение\nстабилизации"(w111) -> ()
        "NoStab" <- FALSE ("NoStab")
      }
    }
  }
  n129 = while {
    shift-right: [w221] -> _
    shift-left: w9 -> [w227]
    stop <- w225 stop-if-true
    # "Еще сюды\nопционально автопилот"
    n130 = local read "Выполняется"() -> (w224:bool)
    n131 = local read "Прервать"() -> (w223:bool)
    n132 = Or(x=w224, y=w223) -> (x .or. y?=w222:bool)
    n133 = case shown="False" w222 {
      tunnel: w227 -> [w228 _]
      tunnel: [w228 "Case"] -> w226
      frame False {
      }
      frame True {
      }
    }
    n134 = case shown="\"Initialization\", Default" w226 {
      tunnel: [_ _ _ _ _ TRUE] -> w225
      tunnel: [w230 w298 w455 w503 w786 T1."Quit" ("Case")] -> w221
      frame "Initialization", Default {
        n135 = stacked-sequence {
          tunnel: [_ _ _ _ T1."TRes_Check(Idle)" ("Case")] -> w230
          frame #0 {
            n136 = property on="Раб. режим LD" class="Bool (strict)"("DisabledEnum"=T3."Enabled" ("Disabled")) -> ()  [unwired: 2 in, 2 out]
          }
          frame #1 {
            # "Питание внешнего фотодиода"
            # "Поменять in0/in1 для ТЕС"
            # "Режим омметра"
            n137 = local read "4070_Rele_source"() -> (w240:enum16{"S2_Ch0", "S1_Ch2"})
            n138 = local read "Source_2_Vcc_out"() -> (w234:refnum<k15>)
            n139 = case shown="\"S2_Ch0\", Default" w240 {
              tunnel: [5.0 -5.0] -> w241
              tunnel: ["0" "2"] -> w242
              tunnel: [w244 w247] -> w243
              frame "S2_Ch0", Default {
                n140 = local read "Source_2_Vcc_out"() -> (w244:refnum<k15>)
              }
              frame "S1_Ch2" {
                n141 = local read "Source_1_Vcc_out"() -> (w247:refnum<k15>)
              }
            }
            n142 = call <instrlib>:"niDCPower Configure Voltage Level.vi"("voltage level"=-5.0, "channel name"="2", "instrument handle"=w234) -> ()  [unwired: 7 in, 2 out]
            n143 = call <instrlib>:"niDCPower Configure Voltage Level.vi"("voltage level"=5.0, "channel name"="1", "instrument handle"=w234) -> ()  [unwired: 7 in, 2 out]
            n144 = call <instrlib>:"niDCPower Configure Voltage Level.vi"("voltage level"=w241, "channel name"=w242, "instrument handle"=w243) -> ()  [unwired: 7 in, 2 out]
            n145 = Wait (ms)(milliseconds to wait=u32 500) -> ()  [unwired: 1 out]
          }
          frame #2 {
            w252 = FALSE
            n146 = local write "NoStab"(w252) -> ()
            n147 = local write "Count_hits?"(w252) -> ()
            n148 = local write "Num_hits"(u64 0 ("Num_hits")) -> ()
            "ThRes_stabil" <- TRUE
            "Boolean 2" <- TRUE
          }
          frame #3 {
            w290 = "\t"
            n149 = local read "Образец"() -> (w270:i32)
            n150 = local read "Температура"() -> (w266:i32)
            n151 = local read "Сеанс"() -> (w261:i32)
            n152 = local read "Ион"() -> (w276:string)
            n153 = Number To Fractional String(number=w270, width (-)=i16 1, precision (6)=i16 0) -> (F-format string=w269:string)  [unwired: 1 in]
            n154 = Number To Fractional String(number=w261, width (-)=i16 1, precision (6)=i16 0) -> (F-format string=w262:string)  [unwired: 1 in]
            n155 = Number To Fractional String(number=w266, width (-)=i16 1, precision (6)=i16 0) -> (F-format string=w265:string)  [unwired: 1 in]
            n156 = Build Path(base path="Param_Log", name or relative path=w276) -> (appended path=w257:path)
            n157 = Build Path(base path=w257, name or relative path="SEL_POM") -> (appended path=w259:path)
            n158 = Concatenate Strings(w269, "_T=" ("string"), w265, "_сеанс" ("string"), w262, ".log" ("string")) -> (w256:string)
            n159 = call <vilib>:"Check if File or Folder Exists.vi"("path"=w259) -> ("file or folder exists?"=w281:bool, "dup path"=w280:path)  [unwired: 8 in, 1 out]
            n160 = case shown="False" w281 {
              tunnel: w280 -> [w295 w296]
              tunnel: [w294 w296] -> w279
              frame False {
                n161 = Create Folder(path (use dialog)=w295) -> (created path=w294:path)  [unwired: 2 in, 2 out]
              }
              frame True {
              }
            }
            n162 = Build Path(base path=w279, name or relative path=w256) -> (appended path=w278:path)
            n163 = Open/Create/Replace File(file path (use dialog)=w278, operation (0:open)=T5."open or create", access (0:read/write)=enum16{"read/write", "read-only", "write-only"}."read/write") -> (refnum out=w260:refnum<file>)  [unwired: 3 in, 2 out]
            n164 = Set File Position(refnum=w260, from (0:start)=enum16{"start", "end", "current"}."end") -> (refnum out=w254:refnum<file>)  [unwired: 2 in, 1 out]
            "refnum out" <- w254
            n165 = Format Into String(initial string=w254, "Time" ("input 1"), w290, "Op_Cur, mA " ("input 6"), w290, "Ipd(EXT), mA", w290, "Im, uA" ("input 6"), w290, "Облучение?", w290, "Превышение тока?", "\r\n") -> (resulting string=w291:refnum<file>)  [unwired: 2 in, 1 out]
            n166 = Set File Position(refnum=w291, from (0:start)=enum16{"start", "end", "current"}."end") -> ()  [unwired: 2 in, 2 out]
          }
          frame #4 {
          }
        }
        n167 = Wait (ms)(milliseconds to wait=u32 100) -> ()  [unwired: 1 out]
        "Status:" <- "Инициализация" ("Status:")
      }
      frame "TEC_Chars" {
        n168 = disable-structure shown="Disabled" {
          disable-tunnel: [w299 _] -> w298
          frame Disabled {
            n169 = while {
              tunnel: [w301] -> w299
              stop <- w300 stop-if-true
              n170 = stacked-sequence {
                tunnel: [_ _ w347 _] -> w301
                tunnel: [_ _ w345 _] -> w300
                frame #0 {
                  n171 = local write "Boolean 2"(FALSE) -> ()
                  n172 = stacked-sequence {
                    frame #0 {
                      # "Переключение в режим Омметра"
                      n173 = local read "4070_Rele_source"() -> (w307:enum16{"S2_Ch0", "S1_Ch2"})
                      n174 = case shown="\"S2_Ch0\", Default" w307 {
                        tunnel: [5.0 -5.0] -> w306
                        tunnel: ["0" "2"] -> w305
                        tunnel: [w308 w311] -> w304
                        frame "S2_Ch0", Default {
                          n175 = local read "Source_2_Vcc_out"() -> (w308:refnum<k15>)
                        }
                        frame "S1_Ch2" {
                          n176 = local read "Source_1_Vcc_out"() -> (w311:refnum<k15>)
                        }
                      }
                      n177 = call <instrlib>:"niDCPower Configure Voltage Level.vi"("voltage level"=w306, "channel name"=w305, "instrument handle"=w304) -> ()  [unwired: 7 in, 2 out]
                    }
                    frame #1 {
                      w314 = FALSE
                      # "Отключение стабилизации"
                      n178 = while {
                        tunnel: w314 -> [_]
                        stop <- w315 stop-if-true
                        n179 = local read "NoStab"() -> (w315:bool)
                      }
                      n180 = local write "ThRes_stabil"(w314) -> ()
                    }
                    frame #2 {
                      # "Перестановка in0 и in1 (+ и - у Пельтье)"
                      n181 = local read "Source_2_Vcc_out"() -> (w317:refnum<k15>)
                      n182 = call <instrlib>:"niDCPower Configure Voltage Level.vi"("voltage level"=-5.0, "channel name"="2", "instrument handle"=w317) -> ()  [unwired: 7 in, 2 out]
                    }
                    frame #3 {
                      # "Отключение пельтье"
                      n183 = local read "Source_1_Vcc_out"() -> (w319:refnum<k15>)
                      n184 = call <instrlib>:"niDCPower Configure Voltage Level.vi"("voltage level"=0.0, "channel name"="2", "instrument handle"=w319) -> ()  [unwired: 7 in, 2 out]
                    }
                    frame #4 {
                      n185 = Wait (ms)(milliseconds to wait="trelax") -> ()  [unwired: 1 out]
                    }
                  }
                  n186 = local write "Status:"("Выравнивание температуры" ("Status:")) -> ()
                }
                frame #1 {
                  w330 = T4 6.5 items=["3 1/2"=3.5, "4 1/2"=4.5, "5 1/2"=5.5, "6 1/2"=6.5, "7 1/2"=7.5] ("Resolution in Digits")
                  n187 = local write "Выполняется"(TRUE) -> ()
                  n188 = local read "4070_address"() -> (w329:refnum<k15>)
                  n189 = call-poly <instrlib>:"niDMM Config Measurement.vi"("Range"=-1.0 ("Configuration:Measurement Options:Max Frequency"), "Resolution in Digits"=w330, "Function"=niDMM_Function."2-wire Resistance" ("multimeter mode"), "instrument handle"=w329) -> ("instrument handle out"=w326:refnum<k15>)  [unwired: 6 in, 1 out]
                  n190 = for {
                    N: 2 -> [_]
                    tunnel: w326 -> [w336]
                    tunnel: [w335] -> w325
                    n191 = call <instrlib>:"niDMM Read.vi"("instrument handle"=w336) -> ("instrument handle out"=w335:refnum<k15>)  [unwired: 8 in, 2 out]
                  }
                  n192 = for {
                    N: 5 -> [_]
                    tunnel: w325 -> [w338]
                    tunnel: [w337] -> w328 mode=indexing
                    n193 = call <instrlib>:"niDMM Read.vi"("instrument handle"=w338) -> ("Measurement"=w337:dbl)  [unwired: 8 in, 2 out]
                    n194 = Wait (ms)(milliseconds to wait=u32 100) -> ()  [unwired: 1 out]
                  }
                  n195 = call-poly <vilib>:"Mean.vi"("X"=w328) -> ("mean"=→"Ro, Ом":dbl)  [unwired: 1 out]
                  n196 = local write "Status:"("Измерение сопротивления в отсутствии тока " ("Status:")) -> ()
                }
                frame #2 {
                  # "Подстройка тока\nдля пельтье"
                  # "При достижении 0V поменять\nполярность, поменяв направление\nтока с помощью реле"
                  n197 = Add(x="Начальное\nнапряжение TEC, В", y="Шаг напр\nдля TEC, В") -> (x+y=w340:dbl)
                  n198 = for {
                    N: "кол-во точек для TEC" -> [_]
                    tunnel: [w370] -> w342 mode=indexing
                    tunnel: [w369] -> w344 mode=indexing
                    tunnel: "Шаг напр\nдля TEC, В" -> [w366]
                    tunnel: [w365] -> w341 mode=indexing
                    shift-right: [w368] -> _
                    shift-left: w340 -> [w367]
                    i -> [w364]
                    # "R"
                    # "I"
                    # "V"
                    n199 = stacked-sequence {
                      seq-local: [w372 _ _] -> [_ w401 _]
                      tunnel: [_ w402 _] -> w369
                      tunnel: [_ _ w430] -> w370
                      tunnel: [_ w401 _] -> w368
                      tunnel: w367 -> [w374 _ _]
                      tunnel: w366 -> [w373 _ _]
                      tunnel: [w371 _ _] -> w365
                      frame #0 {
                        n200 = disable-structure shown="Enabled" {
                          disable-tunnel: w374 -> [w379 w398]
                          disable-tunnel: w373 -> [w378 w399]
                          disable-tunnel: [w377 w397] -> w372
                          disable-tunnel: [w376 w396] -> w371
                          frame Disabled {
                            n201 = local read "кол-во точек для TEC"() -> (w384:i32)
                            n202 = local read item#-1() -> (w381)
                            n203 = Divide(x=w384, y=2) -> (x/y=w382:dbl)
                            n204 = Less?(x=w382, y=w381) -> (x < y?=w380:bool)
                            n205 = case shown="False" w380 {
                              tunnel: [0.0 -5.0] -> w385
                              tunnel: w379 -> [w388 w394]
                              tunnel: w378 -> [w387 w393]
                              tunnel: [w386 w392] -> w377
                              tunnel: [w386 w390] -> w376
                              frame False {
                                n206 = Add(x=w388, y=w387) -> (x+y=w386:dbl)
                              }
                              frame True {
                                n207 = Subtract(x=w394, y=w393) -> (x-y=w392:dbl)
                                n208 = Multiply(x=-1.0, y=w392) -> (x*y=w390:dbl)
                              }
                            }
                          }
                          frame Enabled {
                            n209 = Subtract(x=w398, y=w399) -> (x-y=w397:dbl)
                            n210 = Multiply(x=-1.0, y=w397) -> (x*y=w396:dbl)
                          }
                        }
                        n211 = Wait (ms)(milliseconds to wait=u32 100) -> ()  [unwired: 1 out]
                      }
                      frame #1 {
                        n212 = case shown="\"S1_Ch2\", Default" "TEC_Source" {
                          tunnel: [w425 w427 w429] -> w404
                          tunnel: ["2" "0" "1"] -> w403
                          frame "S1_Ch2", Default {
                            n213 = local read "Source_1_Vcc_out"() -> (w425:refnum<k15>)
                          }
                          frame "S2_Ch0" {
                            n214 = local read "Source_2_Vcc_out"() -> (w427:refnum<k15>)
                          }
                          frame "S3_Ch1" {
                            n215 = local read "Source_3_Vcc_out"() -> (w429:refnum<k15>)
                          }
                        }
                        n216 = flat-sequence {
                          tunnel: [w413] -> w408
                          tunnel: [w410] -> w407
                          tunnel: w404 -> [w412]
                          tunnel: w403 -> [w410]
                          tunnel: w401 -> [w411]
                          tunnel: w408 -> [w414]
                          tunnel: w407 -> [w415]
                          tunnel: [w415] -> w406
                          tunnel: [w414] -> w405
                          tunnel: w406 -> [w420]
                          tunnel: w405 -> [w421]
                          tunnel: [w423] -> w402
                          frame #0 {
                            n217 = call <instrlib>:"niDCPower Configure Voltage Level.vi"("voltage level"=w411, "channel name"=w410, "instrument handle"=w412) -> ("instrument handle out"=w413:refnum<k15>)  [unwired: 7 in, 1 out]
                          }
                          frame #1 {
                            n218 = Wait (ms)(milliseconds to wait=u32 100) -> ()  [unwired: 1 out]
                          }
                          frame #2 {
                            w422 = T6 0 items=["Current", "Voltage"] ("measurement type")
                            n219 = call <instrlib>:"niDCPower Measure.vi"("measurement type"=w422, "channel name"=w420, "instrument handle"=w421) -> ("measurement"=w419:dbl)  [unwired: 6 in, 2 out]
                            n220 = Multiply(x=w419, y=1000.0) -> (x*y=w417:dbl)
                            n221 = Absolute Value(x=w417) -> (abs(x)=w423:dbl)
                            "TEC_current, mA" <- w423
                          }
                        }
                      }
                      frame #2 {
                        w435 = T4 6.5 items=["3 1/2"=3.5, "4 1/2"=4.5, "5 1/2"=5.5, "6 1/2"=6.5, "7 1/2"=7.5] ("Resolution in Digits")
                        # "Снятие показаний\nТерморезистора"
                        n222 = local read "4070_address"() -> (w434:refnum<k15>)
                        n223 = call-poly <instrlib>:"niDMM Config Measurement.vi"("Range"=-1.0 ("Configuration:Measurement Options:Max Frequency"), "Resolution in Digits"=w435, "Function"=niDMM_Function."2-wire Resistance" ("multimeter mode"), "instrument handle"=w434) -> ("instrument handle out"=w433:refnum<k15>)  [unwired: 6 in, 1 out]
                        n224 = for {
                          N: 10 -> [_]
                          tunnel: w433 -> [w439]
                          tunnel: [w438] -> w432 mode=indexing
                          n225 = call <instrlib>:"niDMM Read.vi"("instrument handle"=w439) -> ("Measurement"=w438:dbl)  [unwired: 8 in, 2 out]
                          n226 = Wait (ms)(milliseconds to wait=u32 20) -> ()  [unwired: 1 out]
                        }
                        n227 = call-poly <vilib>:"Mean.vi"("X"=w432) -> ("mean"=w430:dbl)  [unwired: 1 out]
                      }
                    }
                    n228 = Equal?(x=0, y=w364) -> (x = y?=w362:bool)
                    n229 = Select(t=u32 3000, s=w362, f="milliseconds to wait") -> (s? t:f=w361:u32)
                    n230 = Wait (ms)(milliseconds to wait=w361) -> ()  [unwired: 1 out]
                  }
                  n231 = local write "Status:"("Построение характеристики TEC" ("Status:")) -> ()
                  n232 = flat-sequence {
                    tunnel: [T1."TRes_Check(Idle)" ("Case")] -> w347
                    tunnel: w344 -> [w356]
                    tunnel: [TRUE] -> w345
                    tunnel: w342 -> [w354]
                    tunnel: w342 -> [w352]
                    tunnel: w341 -> [w351]
                    frame #0 {
                      # "Построение харак-ки TEC\nи опциональная запись"
                      n233 = Bundle(w356, w354) -> (→"RES(I_TEC) Graph":cluster{dbl[], dbl[]})  [unwired: 1 in]
                      n234 = Bundle(w351, w352) -> (→"RES(U_TEC) Graph":cluster{dbl[], dbl[]})  [unwired: 1 in]
                      n235 = local write "Выполняется"(FALSE) -> ()
                    }
                  }
                }
                frame #3 {
                  n236 = disable-structure shown="Disabled" {
                    frame Disabled {
                      # "Переключение в режим Вольтметра"
                      n237 = local read "4070_Rele_source"() -> (w443:enum16{"S2_Ch0", "S1_Ch2"})
                      n238 = case shown="\"S2_Ch0\", Default" w443 {
                        tunnel: [0.0 0.0] -> w446
                        tunnel: ["0" "2"] -> w445
                        tunnel: [w447 w450] -> w444
                        frame "S2_Ch0", Default {
                          n239 = local read "Source_2_Vcc_out"() -> (w447:refnum<k15>)
                        }
                        frame "S1_Ch2" {
                          n240 = local read "Source_1_Vcc_out"() -> (w450:refnum<k15>)
                        }
                      }
                      n241 = call <instrlib>:"niDCPower Configure Voltage Level.vi"("voltage level"=w446, "channel name"=w445, "instrument handle"=w444) -> ()  [unwired: 7 in, 2 out]
                    }
                    frame Enabled {
                    }
                  }
                  n242 = Wait (ms)(milliseconds to wait=u32 1000) -> ()  [unwired: 1 out]
                  n243 = local write "ThRes_stabil"(TRUE) -> ()
                }
              }
            }
          }
          frame Enabled {
          }
        }
      }
      frame "TRes_Check(Idle)" {
        n244 = flat-sequence {
          tunnel: [w477] -> w457
          tunnel: [w479] -> w456
          tunnel: w457 -> [w480]
          tunnel: w456 -> [w482]
          tunnel: [w481] -> w453
          tunnel: [w502] -> w455
          tunnel: w453 -> [w502]
          frame #0 {
            w467 = i16 3 ("width (-)")
            w461 = "\t"
            w474 = i16 3 ("width (-)")
            w475 = i16 3 ("width (-)")
            n245 = local read "refnum out"() -> (w479:refnum<file>)
            n246 = local read "Operating Current, mA"() -> (w460:dbl)
            n247 = local read "I_pd, uA"() -> (w458:dbl)
            n248 = local read "IPD(ext), mA"() -> (w473:dbl)
            n249 = Select(t="Облучение", s="Облучение!", f="") -> (s? t:f=w462:string)
            n250 = Get Date/Time In Seconds() -> (seconds since 1Jan1904=w471:timestamp)
            n251 = Format Date/Time String(time format string (%c)="%d  %H:%M:%S", seconds (now)=w471) -> (date/time string=w470:string)  [unwired: 1 in]
            n252 = Number To Fractional String(number=w460, width (-)=w475, precision (6)=w475) -> (F-format string=w469:string)  [unwired: 1 in]
            n253 = Number To Fractional String(number=w473, width (-)=w474, precision (6)=w474) -> (F-format string=w468:string)  [unwired: 1 in]
            n254 = Number To Fractional String(number=w458, width (-)=w467, precision (6)=w467) -> (F-format string=w466:string)  [unwired: 1 in]
            n255 = Greater?(x=w460, y="Порог типатиристора, мА") -> (0:w478:bool)
            n256 = Format Into String(initial string=w479, w470, w461, w469, w461, w468, w461, w466, w461, w462, w461) -> ()  [unwired: 2 in, 2 out]
            n257 = Or(x="SEL simulation", y=w478) -> (x .or. y?=w477:bool)
          }
          frame #1 {
            n258 = case shown="True" w480 {
              tunnel: ["" w487] -> w484
              tunnel: [T1."TRes_Check(Idle)" ("Case") w488] -> w481
              frame False {
              }
              frame True {
                n259 = stacked-sequence {
                  tunnel: [_ _ T1."TRes_Check(Idle)" ("Case")] -> w488
                  tunnel: [_ _ "!!!!"] -> w487
                  frame #0 {
                    n260 = local read "Source_1_Vcc_out"() -> (w490:refnum<k15>)
                    n261 = call <instrlib>:"niDCPower Configure Voltage Level.vi"("voltage level"=0.0, "channel name"="0", "instrument handle"=w490) -> ()  [unwired: 7 in, 2 out]
                  }
                  frame #1 {
                    n262 = Wait (ms)(milliseconds to wait="milliseconds to wait 2") -> ()  [unwired: 1 out]
                  }
                  frame #2 {
                    n263 = local read "accommodated voltage (out)"() -> (w494:dbl)
                    n264 = local read "Счетчик сбоев"() -> (w497:dbl)
                    n265 = local read "Source_1_Vcc_out"() -> (w495:refnum<k15>)
                    n266 = Increment(x=w497) -> (x+1=w498:dbl)
                    n267 = local write "Счетчик сбоев"(w498) -> ()
                    n268 = call <instrlib>:"niDCPower Configure Voltage Level.vi"("voltage level"=w494, "channel name"="0", "instrument handle"=w495) -> ()  [unwired: 7 in, 2 out]
                    n269 = local write "SEL simulation"(FALSE) -> ()
                  }
                }
              }
            }
            n270 = Format Into String(initial string=w482, w484, "\r\n") -> ()  [unwired: 2 in, 2 out]
          }
          frame #2 {
            n271 = Wait (ms)(milliseconds to wait=u32 250) -> ()  [unwired: 1 out]
          }
        }
        n272 = local write "Status:"("IDLE" ("Status:")) -> ()
      }
      frame "Characteristics" {
        n273 = disable-structure shown="Disabled" {
          disable-tunnel: [w505 _] -> w503
          frame Disabled {
            n274 = flat-sequence {
              tunnel: [w523] -> w516
              tunnel: [w527] -> w515
              tunnel: [w526] -> w514
              tunnel: [w525] -> w513
              tunnel: [w522] -> w512
              tunnel: [w520] -> w511
              tunnel: w516 -> [w757]
              tunnel: [w757] -> w510
              tunnel: w515 -> [w742]
              tunnel: [w742] -> w509
              tunnel: w514 -> [w759]
              tunnel: [w759] -> w508
              tunnel: w513 -> [w743]
              tunnel: [w743] -> w507
              tunnel: w512 -> [w758]
              tunnel: [w758] -> w506
              tunnel: w511 -> [w733]
              tunnel: [T1."TRes_Check(Idle)" ("Case")] -> w505
              tunnel: w510 -> [w760]
              tunnel: w509 -> [w780]
              tunnel: w508 -> [w779]
              tunnel: w507 -> [w777]
              tunnel: w506 -> [w774]
              frame #0 {
                n275 = local read "Отладка(F)/\n/Рабочий(T)"() -> (w517:bool)
                n276 = case shown="True" w517 {
                  frame False {
                  }
                  frame True {
                    n277 = while {
                      stop <- w519 stop-if-true
                      n278 = call "Save_dialogue_dose.vi"() -> ("output 1"=w518:dbl)  [unwired: 11 in]
                      n279 = Not Equal To 0?(x=w518) -> (x != 0?=w519:bool)
                    }
                  }
                }
              }
              frame #1 {
                # "Хар-ки:\nI_LD (V);\nOphir(I_LD);\nI_PD(I_LD);\nRcheck(I_LD)"
                n280 = Subtract(x="Начальный ток, мА", y="Шаг, мА") -> (x-y=w528:dbl)
                n281 = for {
                  N: "Кол-во точек" -> [_]
                  shift-right: [w537] -> _
                  shift-left: w528 -> [w539]
                  tunnel: [w537] -> w523 mode=indexing
                  tunnel: [w536] -> w527 mode=indexing
                  tunnel: [w535] -> w526 mode=indexing
                  tunnel: [w534] -> w525 mode=indexing
                  tunnel: [w532] -> w522 mode=indexing
                  tunnel: [w530] -> w520
                  i -> [w533]
                  # "ExtPD"
                  # "FV"
                  # "I_PD"
                  # "I_LD"
                  # "Ophir"
                  n282 = property on="Шаг, мА" class="DigNum (strict)"() -> ("Value"=w531:dbl)  [unwired: 2 in, 2 out]
                  n283 = Add(x=w539, y=w531) -> (x+y=w538:dbl)
                  n284 = stacked-sequence {
                    tunnel: w538 -> [_ w560 _ _ _ _ _ _ _]
                    tunnel: [_ w554 _ _ _ _ _ _ _] -> w537
                    tunnel: [_ _ _ _ _ w623 _ _ _] -> w536
                    tunnel: [_ _ _ _ _ _ w639 _ _] -> w535
                    tunnel: [_ _ _ _ w614 _ _ _ _] -> w534
                    tunnel: w533 -> [_ _ _ _ _ _ _ _ w676]
                    tunnel: [_ _ _ _ _ _ _ w652 _] -> w532
                    tunnel: [_ _ _ _ _ _ _ _ w675] -> w530
                    frame #0 {
                      n285 = disable-structure shown="Disabled" {
                        frame Disabled {
                          n286 = stacked-sequence {
                            frame #0 {
                              w540 = FALSE
                              # "Отключение стабилизации"
                              n287 = while {
                                tunnel: w540 -> [_]
                                stop <- w541 stop-if-true
                                n288 = local read "NoStab"() -> (w541:bool)
                              }
                              n289 = local write "ThRes_stabil"(w540) -> ()
                            }
                            frame #1 {
                              # "Переключение в режим Вольтметра"
                              n290 = local read "4070_Rele_source"() -> (w542:enum16{"S2_Ch0", "S1_Ch2"})
                              n291 = case shown="\"S2_Ch0\", Default" w542 {
                                tunnel: [0.0 0.0] -> w545
                                tunnel: ["0" "2"] -> w544
                                tunnel: [w546 w549] -> w543
                                frame "S2_Ch0", Default {
                                n292 = local read "Source_2_Vcc_out"() -> (w546:refnum<k15>)
                                }
                                frame "S1_Ch2" {
                                n293 = local read "Source_1_Vcc_out"() -> (w549:refnum<k15>)
                                }
                              }
                              n294 = call <instrlib>:"niDCPower Configure Voltage Level.vi"("voltage level"=w545, "channel name"=w544, "instrument handle"=w543) -> ()  [unwired: 7 in, 2 out]
                            }
                          }
                        }
                        frame Enabled {
                        }
                      }
                    }
                    frame #1 {
                      # "Подстройка тока\nлазерного диода"
                      n295 = local read "Source_1_Vcc_out"() -> (w561:refnum<k15>)
                      n296 = disable-structure shown="Enabled" {
                        disable-tunnel: "the lower limit for the voltage_LD" -> [w578 w584]
                        disable-tunnel: "Start voltage_LD" -> [w577 w585]
                        disable-tunnel: "the upper limit for the voltage_LD" -> [w576 w586]
                        disable-tunnel: w561 -> [w575 w583]
                        disable-tunnel: w560 -> [w574 w582]
                        disable-tunnel: "Res_LD" -> [w573 w581]
                        disable-tunnel: "0" -> [w572 w579]
                        disable-tunnel: "accuracy_LD" -> [w571 w589]
                        disable-tunnel: [w570 w588] -> w556
                        disable-tunnel: [w568 w587] -> w555
                        disable-tunnel: [w567 w580] -> w554
                        frame Disabled {
                          n297 = local read "4070_address"() -> (w569:refnum<k15>)
                          n298 = call "Set input current_ChAmmeter.vi"("the lower limit for the voltage"=w578, "accuracy (input)"=w571, "4070_address"=w569, "Start voltage"=w577, "the upper limit for the voltage"=w576, "instrument handle"=w575, "the optimum current(input)"=w574, "res(input)"=w573, "channel name"=w572) -> ("accommodated voltage (out)"=w570:dbl, "current value, mA"=w567:dbl, "the voltage drop across the resistor"=w568:dbl)  [unwired: 3 in, 1 out]
                        }
                        frame Enabled {
                          n299 = call "Set input current_ChSource.vi"("channel name"=w579, "res(input)"=w581, "the optimum current(input)"=w582, "accuracy (input)"=w589, "instrument handle"=w583, "the upper limit for the voltage"=w586, "Start voltage"=w585, "the lower limit for the voltage"=w584) -> ("current value, mA"=w580:dbl, "the voltage drop across the resistor"=w587:dbl, "accommodated voltage (out)"=w588:dbl)  [unwired: 1 out]
                        }
                      }
                      "Подстроенный ток, mA" <- w554
                      "accommodated voltage (out)" <- w556
                      "Volt_onRes" <- w555
                      n300 = local write "Status:"("Подстройка тока LD" ("Status:")) -> ()
                      n301 = Wait (ms)(milliseconds to wait=u32 100) -> ()  [unwired: 1 out]
                      n302 = Greater Or Equal?(x=w554, y=49.5) -> (x >= y?=→"Boolean":bool)
                    }
                    frame #2 {
                      # "and stab"
                      # "Resistance check"
                      n303 = flat-sequence {
                        frame #0 {
                          n304 = disable-structure shown="Disabled" {
                            frame Disabled {
                              # "Режим Омметра"
                              n305 = case shown="\"S2_Ch0\", Default" "4070_Rele_source" {
                                tunnel: [5.0 -5.0] -> w593
                                tunnel: ["0" "2"] -> w592
                                tunnel: [w595 w598] -> w591
                                frame "S2_Ch0", Default {
                                n306 = local read "Source_2_Vcc_out"() -> (w595:refnum<k15>)
                                }
                                frame "S1_Ch2" {
                                n307 = local read "Source_1_Vcc_out"() -> (w598:refnum<k15>)
                                }
                              }
                              n308 = call <instrlib>:"niDCPower Configure Voltage Level.vi"("voltage level"=w593, "channel name"=w592, "instrument handle"=w591) -> ()  [unwired: 7 in, 2 out]
                            }
                            frame Enabled {
                            }
                          }
                        }
                        frame #1 {
                          n309 = Wait (ms)(milliseconds to wait=u32 1000) -> ()  [unwired: 1 out]
                          "Num_hits" <- u64 0 ("Num_hits")
                        }
                        frame #2 {
                          n310 = local write "ThRes_stabil"(TRUE) -> ()
                        }
                        frame #3 {
                          n311 = local write "Count_hits?"(TRUE ("Acq_allow?")) -> ()
                          n312 = Wait (ms)(milliseconds to wait="tstab между точками, мс") -> ()  [unwired: 1 out]
                        }
                      }
                      n313 = local write "Status:"("Проверка и стабилизация сопротивления" ("Status:")) -> ()
                    }
                    frame #3 {
                      n314 = while {
                        tunnel: [u64 0] -> w607
                        tunnel: [FALSE ("Acq_allow?")] -> w606
                        stop <- w610 stop-if-true
                        n315 = local read "Num_hits"() -> (w612:u64)
                        n316 = Greater Or Equal?(x=w612, y="Num_hits_req") -> (x >= y?=w610:bool)
                      }
                      n317 = local write "Count_hits?"(w606) -> ()
                      n318 = local write "Num_hits"(w607) -> ()
                    }
                    frame #4 {
                      # "Forward\nVoltage\nmeasurement"
                      n319 = local read "Source_1_Vcc_out"() -> (w620:refnum<k15>)
                      n320 = local read "Volt_onRes"() -> (w613:dbl)
                      n321 = call <instrlib>:"niDCPower Measure Multiple.vi"("channel name"="0", "instrument handle"=w620) -> ("voltage measurements"=w618:dbl[])  [unwired: 6 in, 3 out]
                      n322 = Index Array(array=w618) -> (element=w616:dbl)  [unwired: 1 in]
                      n323 = Absolute Value(x=w613) -> (abs(x)=w615:dbl)
                      n324 = Absolute Value(x=w616) -> (abs(x)=w617:dbl)
                      n325 = Subtract(x=w617, y=w615) -> (x-y=w614:dbl)
                      "Forward Voltage, V" <- w614
                      n326 = local write "Status:"("Измерение прямого напряжения" ("Status:")) -> ()
                      n327 = Wait (ms)(milliseconds to wait=u32 100) -> ()  [unwired: 1 out]
                    }
                    frame #5 {
                      # "Ophir\nmeasurement"
                      n328 = property on="Ophir_address" class="Ref (strict)"() -> ("Value"=w625:refnum<k7>)  [unwired: 2 in, 2 out]
                      n329 = property on="hDevice" class="DigNum (strict)"() -> ("Value"=w624:i32)  [unwired: 2 in, 2 out]
                      n330 = invoke class="ICoLMMeasurement" method="GetData"(reference=w625, "hDevice"=w624, "channel"=0) -> ("arrayValue"=w632:variant)  [unwired: 5 in, 7 out]
                      n331 = local write "Status:"("Измерен. оптич. мощности" ("Status:")) -> ()
                      n332 = Variant To Data(type=dbl[] [], Variant=w632) -> (data=w629:dbl[])  [unwired: 1 in, 1 out]
                      n333 = Wait (ms)(milliseconds to wait=u32 200) -> ()  [unwired: 1 out]
                      n334 = Array Size(array=w629) -> (size(s)=w627:i32)
                      n335 = Decrement(x=w627) -> (x-1=w626:i32)
                      n336 = Index Array(array=w629, index=w626) -> (element=w628:dbl)
                      n337 = Multiply(x=1000.0, y=w628) -> (x*y=w623:dbl)
                      "Ophir, mW" <- w623
                    }
                    frame #6 {
                      w642 = T4 7.5 items=["3 1/2"=3.5, "4 1/2"=4.5, "5 1/2"=5.5, "6 1/2"=6.5, "7 1/2"=7.5] ("Resolution in Digits")
                      # "Inside I_PD\nmeasurements"
                      n338 = local read "4071(1)_adress"() -> (w643:refnum<k15>)
                      n339 = call-poly <instrlib>:"niDMM Config Measurement.vi"("Range"=-1.0 ("Configuration:Measurement Options:Max Frequency"), "Resolution in Digits"=w642, "Function"=niDMM_Function."DC Current" ("multimeter mode"), "instrument handle"=w643) -> ("instrument handle out"=w641:refnum<k15>)  [unwired: 6 in, 1 out]
                      n340 = for {
                        N: 5 -> [_]
                        tunnel: w641 -> [w650]
                        tunnel: [w647] -> w636 mode=indexing
                        n341 = call <instrlib>:"niDMM Read.vi"("instrument handle"=w650) -> ("Measurement"=w648:dbl)  [unwired: 8 in, 2 out]
                        n342 = Absolute Value(x=w648) -> (abs(x)=w647:dbl)
                        n343 = Wait (ms)(milliseconds to wait=u32 50) -> ()  [unwired: 1 out]
                      }
                      n344 = local write "Status:"("I_PD встроенного фотодиода" ("Status:")) -> ()
                      n345 = call-poly <vilib>:"Mean.vi"("X"=w636) -> ("mean"=w637:dbl)  [unwired: 1 out]
                      n346 = Multiply(x=w637, y=1000000.0) -> (x*y=w639:dbl)
                      "I_pd, uA" <- w639
                    }
                    frame #7 {
                      # "EXTERNAL I_PD\nmeasurements"
                      n347 = disable-structure shown="Enabled" {
                        disable-tunnel: [w655 w670] -> w652
                        disable-tunnel: [_ w670] -> w651
                        frame Disabled {
                          w662 = T4 6.5 items=["3 1/2"=3.5, "4 1/2"=4.5, "5 1/2"=5.5, "6 1/2"=6.5, "7 1/2"=7.5] ("Resolution in Digits")
                          n348 = local read "4071(2)_adress"() -> (w663:refnum<k15>)
                          n349 = call-poly <instrlib>:"niDMM Config Measurement.vi"("Range"=-1.0 ("Configuration:Measurement Options:Max Frequency"), "Resolution in Digits"=w662, "Function"=niDMM_Function."DC Current" ("multimeter mode"), "instrument handle"=w663) -> ("instrument handle out"=w661:refnum<k15>)  [unwired: 6 in, 1 out]
                          n350 = for {
                            N: 5 -> [_]
                            tunnel: w661 -> [w668]
                            tunnel: [w666] -> w659 mode=indexing
                            n351 = call <instrlib>:"niDMM Read.vi"("instrument handle"=w668) -> ("Measurement"=w666:dbl)  [unwired: 8 in, 2 out]
                            n352 = Wait (ms)(milliseconds to wait=u32 50) -> ()  [unwired: 1 out]
                          }
                          n353 = call-poly <vilib>:"Mean.vi"("X"=w659) -> ("mean"=w658:dbl)  [unwired: 1 out]
                          n354 = Absolute Value(x=w658) -> (abs(x)=w657:dbl)
                          n355 = Multiply(x=w657, y=1000.0) -> (x*y=w655:dbl)
                        }
                        frame Enabled {
                          n356 = local read "Source_2_Vcc_out"() -> (w674:refnum<k15>)
                          n357 = call <instrlib>:"niDCPower Measure Multiple.vi"("channel name"="1", "instrument handle"=w674) -> ("current measurements"=w672:dbl[])  [unwired: 6 in, 3 out]
                          n358 = Index Array(array=w672) -> (element=w669:dbl)  [unwired: 1 in]
                          n359 = Multiply(x=w669, y=1000.0) -> (x*y=w670:dbl)
                        }
                      }
                      "IPD(ext), mA" <- w651
                      n360 = local write "Status:"("I_PD внешнего фотодиода" ("Status:")) -> ()
                      n361 = Wait (ms)(milliseconds to wait=u32 200) -> ()  [unwired: 1 out]
                    }
                    frame #8 {
                      n362 = local read "Отладка(F)/\n/Рабочий(T)"() -> (w677:bool)
                      n363 = case shown="True" w677 {
                        tunnel: w676 -> [_ w696]
                        tunnel: [_ w678] -> w675
                        frame False {
                        }
                        frame True {
                          w686 = i16 3 ("width (-)")
                          w687 = i16 3 ("width (-)")
                          w689 = i16 3 ("width (-)")
                          w692 = i16 3 ("width (-)")
                          w695 = i16 3 ("width (-)")
                          # "Внешний ФД"
                          # "Офир"
                          n364 = local read "IPD(ext), mA"() -> (w680:dbl)
                          n365 = local read "Ophir, mW"() -> (w679:dbl)
                          n366 = local read "Forward Voltage, V"() -> (w691:dbl)
                          n367 = local read "Подстроенный ток, mA"() -> (w694:dbl)
                          n368 = local read "I_pd, uA"() -> (w688:dbl)
                          n369 = Equal To 0?(x=w696) -> (x = 0?=w684:bool)
                          n370 = Number To Fractional String(number=w694, width (-)=w695, precision (6)=w695) -> (F-format string=w693:string)  [unwired: 1 in]
                          n371 = Number To Fractional String(number=w691, width (-)=w692, precision (6)=w692) -> (F-format string=w690:string)  [unwired: 1 in]
                          n372 = Number To Fractional String(number=w680, width (-)=w689, precision (6)=w689) -> (F-format string=w681:string)  [unwired: 1 in]
                          n373 = Number To Fractional String(number=w688, width (-)=w687, precision (6)=w687) -> (F-format string=w682:string)  [unwired: 1 in]
                          n374 = Number To Fractional String(number=w679, width (-)=w686, precision (6)=w686) -> (F-format string=w683:string)  [unwired: 1 in]
                          n375 = case shown="True" w684 {
                            tunnel: ["" ("date/time string") w701] -> w678
                            tunnel: ["" w699] -> w685
                            frame False {
                            }
                            frame True {
                              w700 = i16 0 ("width (-)")
                              n376 = Get Date/Time In Seconds() -> (seconds since 1Jan1904=w703:timestamp)
                              n377 = Format Date/Time String(time format string (%c)="%d  %H:%M:%S", seconds (now)=w703) -> (date/time string=w701:string)  [unwired: 1 in]
                              n378 = Number To Fractional String(width (-)=w700, precision (6)=w700) -> (F-format string=w699:string)  [unwired: 2 in]
                            }
                          }
                          n379 = stacked-sequence {
                            tunnel: w678 -> [w710 w718 w725 _ w732]
                            tunnel: w685 -> [w709 w715 w723 _ w731]
                            tunnel: w693 -> [w707 w714 w722 _ w727]
                            tunnel: w690 -> [w705 _ _ _ _]
                            tunnel: w683 -> [_ w713 _ _ _]
                            tunnel: w682 -> [_ _ w720 _ _]
                            tunnel: w681 -> [_ _ _ _ w729]
                            frame #0 {
                              w706 = "\t"
                              n380 = Format Into String(w710, w706, "", w706, w709, w706, w707, w706, w705, "\r\n") -> ()  [unwired: 3 in, 2 out]
                            }
                            frame #1 {
                              w712 = "\t"
                              n381 = local read item#-1() -> (w717)
                              n382 = Format Into String(initial string=w717, w718, w712, "", w712, w715, w712, w714, w712, w713, "\r\n") -> ()  [unwired: 2 in, 2 out]
                            }
                            frame #2 {
                              w721 = "\t"
                              n383 = Format Into String(w725, w721, "", w721, w723, w721, w722, w721, w720, "\r\n") -> ()  [unwired: 3 in, 2 out]
                            }
                            frame #3 {
                            }
                            frame #4 {
                              w728 = "\t"
                              n384 = Format Into String(w732, w728, "", w728, w731, w728, w727, w728, w729, "\r\n") -> ()  [unwired: 3 in, 2 out]
                            }
                          }
                        }
                      }
                    }
                  }
                }
              }
              frame #2 {
                w739 = i16 3 ("width (-)")
                w745 = i16 3 ("width (-)")
                w747 = i16 3 ("width (-)")
                w750 = i16 3 ("width (-)")
                w752 = "" ("input 1")
                w737 = "\t"
                w755 = i16 3 ("width (-)")
                # "Рабочее напряжение"
                n385 = local read "Подстроенный ток, mA"() -> (w749:dbl)
                n386 = local read "Ophir, mW"() -> (w744:dbl)
                n387 = call "Find_ThresholdOphir_F4.vi"("Threshold Ophir"=5.0, "Current array"=w743, "Ophir array"=w742) -> ("Threshold Current"=w740:dbl)  [unwired: 8 in]
                n388 = call "Find_ThresholdOphir_F4.vi"("Threshold Ophir"=1.0, "Current array"=w757, "Ophir array"=w742) -> ("Threshold Current"=w754:dbl)  [unwired: 8 in]
                "Пороговый ток" <- w754
                n389 = local read "I_pd, uA"() -> (w738:dbl)
                n390 = Number To Fractional String(number=w740, width (-)=w747, precision (6)=w747) -> (F-format string=w746:string)  [unwired: 1 in]
                n391 = Number To Fractional String(number=w754, width (-)=w755, precision (6)=w755) -> (F-format string=w751:string)  [unwired: 1 in]
                n392 = Number To Fractional String(number=w738, width (-)=w739, precision (6)=w739) -> (F-format string=w735:string)  [unwired: 1 in]
                n393 = Number To Fractional String(number=w744, width (-)=w745, precision (6)=w745) -> (F-format string=w734:string)  [unwired: 1 in]
                n394 = Number To Fractional String(number=w749, width (-)=w750, precision (6)=w750) -> (F-format string=w748:string)  [unwired: 1 in]
                n395 = Format Into String(w733, w737, w752, w737, w752, w737, w751, w737, w748, w737, w746, w737, w735, w737, w734, "\r\n") -> (initial string=w753:refnum<file>)  [unwired: 2 in, 2 out]
              }
              frame #3 {
                n396 = property on="Boolean" class="Bool (strict)"() -> ("Value"=w769:bool)  [unwired: 2 in, 2 out]
                n397 = And(x=w769, y="Оставить в раб.\nрежиме") -> (x .and. y?=w770:bool)
                n398 = local read "Source_1_Vcc_out"() -> (w772:refnum<k15>)
                n399 = local read "Подстроенное напряжение\nстабилизации"() -> (w766:dbl)
                n400 = case shown="True" w770 {
                  tunnel: [0.0 ("voltage level") w785] -> w771
                  frame False {
                  }
                  frame True {
                    n401 = local read "accommodated voltage (out)"() -> (w785:dbl)
                  }
                }
                n402 = local read "Source_1_Vcc_out"() -> (w765:refnum<k15>)
                n403 = Bundle(w760, w780) -> (→"OP(I_LD) Graph":cluster{dbl[], dbl[]})  [unwired: 1 in]
                n404 = Bundle(w760, w779) -> (→"I_PD(I_LD) Graph":cluster{dbl[], dbl[]})  [unwired: 1 in]
                n405 = Bundle(w760, w777) -> (→"V2(I_LD) Graph":cluster{dbl[], dbl[]})  [unwired: 1 in]
                n406 = Bundle(w760, w774) -> (→"I_PD_Ext(I_LD) Graph":cluster{dbl[], dbl[]})  [unwired: 1 in]
                n407 = Add(x=w766, y=0.2) -> (x+y=w761:dbl)
                n408 = local write "Выполняется"(FALSE) -> ()
                n409 = Multiply(x=w761, y=-1.0) -> (x*y=w762:dbl)
                n410 = call <instrlib>:"niDCPower Configure Voltage Level.vi"("voltage level"=w762, "channel name"="2", "instrument handle"=w765) -> ()  [unwired: 7 in, 2 out]
                n411 = call <instrlib>:"niDCPower Configure Voltage Level.vi"("voltage level"=w771, "channel name"="0", "instrument handle"=w772) -> ()  [unwired: 7 in, 2 out]
              }
            }
            n412 = local write "Boolean 2"(FALSE) -> ()
          }
          frame Enabled {
          }
        }
      }
      frame "Bias" {
        n413 = local write "Boolean 2"(FALSE) -> ()
        n414 = stacked-sequence {
          tunnel: [_ _ _ _ w853] -> w786
          frame #0 {
            n415 = disable-structure shown="Disabled" {
              frame Disabled {
                w789 = FALSE
                n416 = while {
                  tunnel: w789 -> [_]
                  stop <- w790 stop-if-true
                  n417 = local read "NoStab"() -> (w790:bool)
                }
                n418 = local write "ThRes_stabil"(w789) -> ()
              }
              frame Enabled {
              }
            }
            n419 = local write "Num_hits"(0) -> ()
          }
          frame #1 {
            n420 = disable-structure shown="Disabled" {
              frame Disabled {
                # "Переключение в режим Вольтметра"
                n421 = local read "4070_Rele_source"() -> (w791:enum16{"S2_Ch0", "S1_Ch2"})
                n422 = case shown="\"S2_Ch0\", Default" w791 {
                  tunnel: [0.0 0.0] -> w794
                  tunnel: ["0" "2"] -> w793
                  tunnel: [w795 w798] -> w792
                  frame "S2_Ch0", Default {
                    n423 = local read "Source_2_Vcc_out"() -> (w795:refnum<k15>)
                  }
                  frame "S1_Ch2" {
                    n424 = local read "Source_1_Vcc_out"() -> (w798:refnum<k15>)
                  }
                }
                n425 = call <instrlib>:"niDCPower Configure Voltage Level.vi"("voltage level"=w794, "channel name"=w793, "instrument handle"=w792) -> ()  [unwired: 7 in, 2 out]
              }
              frame Enabled {
              }
            }
          }
          frame #2 {
            n426 = local read "the upper limit for the voltage_LD"() -> (w816:dbl)
            n427 = local read "the lower limit for the voltage_LD"() -> (w818:dbl)
            n428 = local read "Source_1_Vcc_out"() -> (w815:refnum<k15>)
            n429 = local read "Start voltage_LD"() -> (w817:dbl)
            n430 = local read "accuracy_LD"() -> (w812:dbl)
            n431 = local read "Res_LD"() -> (w814:dbl)
            n432 = disable-structure shown="Enabled" {
              disable-tunnel: "Desirable Operating current, mA" -> [w830 w836]
              disable-tunnel: [w829 w837] -> w801
              disable-tunnel: w818 -> [w828 w840]
              disable-tunnel: w817 -> [w827 w831]
              disable-tunnel: w816 -> [w826 w832]
              disable-tunnel: w815 -> [w825 w833]
              disable-tunnel: w814 -> [w824 w835]
              disable-tunnel: "0" ("channel name") -> [w823 w834]
              disable-tunnel: w812 -> [w822 w839]
              disable-tunnel: [w821 w838] -> w811
              frame Disabled {
                n433 = local read "4070_address"() -> (w820:refnum<k15>)
                n434 = call "Set input current_ChAmmeter.vi"("the lower limit for the voltage"=w828, "accuracy (input)"=w822, "4070_address"=w820, "Start voltage"=w827, "the upper limit for the voltage"=w826, "instrument handle"=w825, "the optimum current(input)"=w830, "res(input)"=w824, "channel name"=w823) -> ("accommodated voltage (out)"=w821:dbl, "current value, mA"=w829:dbl)  [unwired: 3 in, 2 out]
              }
              frame Enabled {
                n435 = call "Set input current_ChSource.vi"("channel name"=w834, "res(input)"=w835, "the optimum current(input)"=w836, "accuracy (input)"=w839, "instrument handle"=w833, "the upper limit for the voltage"=w832, "Start voltage"=w831, "the lower limit for the voltage"=w840) -> ("current value, mA"=w837:dbl, "accommodated voltage (out)"=w838:dbl)  [unwired: 2 out]
              }
            }
            "Operating Current, mA" <- w801
            n436 = local read "+ V TEC для новой точки"() -> (w806:dbl)
            n437 = local read "Подстроенное напряжение\nстабилизации"() -> (w804:dbl)
            n438 = local write "Подстроенный ток, mA"(w801) -> ()
            n439 = local read "Source_1_Vcc_out"() -> (w810:refnum<k15>)
            n440 = local write "accommodated voltage (out)"(w811) -> ()
            n441 = Multiply(x=w806, y=2.0) -> (x*y=w803:dbl)
            n442 = Add(x=w803, y=w804) -> (x+y=w802:dbl)
            n443 = Multiply(x=w802, y=-1.0) -> (x*y=w807:dbl)
            n444 = call <instrlib>:"niDCPower Configure Voltage Level.vi"("voltage level"=w807, "channel name"="2", "instrument handle"=w810) -> ()  [unwired: 7 in, 2 out]
          }
          frame #3 {
            n445 = disable-structure shown="Enabled" {
              frame Disabled {
                # "Переключение в режим Омметра"
                n446 = local read "4070_Rele_source"() -> (w846:enum16{"S2_Ch0", "S1_Ch2"})
                n447 = case shown="\"S2_Ch0\", Default" w846 {
                  tunnel: [5.0 -5.0] -> w845
                  tunnel: ["0" "2"] -> w844
                  tunnel: [w847 w850] -> w843
                  frame "S2_Ch0", Default {
                    n448 = local read "Source_2_Vcc_out"() -> (w847:refnum<k15>)
                  }
                  frame "S1_Ch2" {
                    n449 = local read "Source_1_Vcc_out"() -> (w850:refnum<k15>)
                  }
                }
                n450 = call <instrlib>:"niDCPower Configure Voltage Level.vi"("voltage level"=w845, "channel name"=w844, "instrument handle"=w843) -> ()  [unwired: 7 in, 2 out]
              }
              frame Enabled {
              }
            }
            n451 = local write "Выполняется"(FALSE) -> ()
            n452 = local write "ThRes_stabil"(TRUE) -> ()
          }
          frame #4 {
            n453 = flat-sequence {
              tunnel: [T1."TRes_Check(Idle)" ("Case")] -> w853
              frame #0 {
                n454 = Wait (ms)(milliseconds to wait=u32 3000) -> ()  [unwired: 1 out]
              }
              frame #1 {
                n455 = disable-structure shown="Enabled" {
                  disable-tunnel: [w856 w868] -> w855
                  frame Disabled {
                    n456 = local read "Operating Current, mA"() -> (w859:dbl)
                    n457 = Greater Or Equal?(x=w859, y=45.0) -> (x >= y?=w857:bool)
                    n458 = disable-structure shown="Enabled" {
                      disable-tunnel: w857 -> [w861 w867]
                      disable-tunnel: [w860 w867] -> w856
                      frame Disabled {
                        n459 = case shown="True" w861 {
                          tunnel: [FALSE w863] -> w860
                          frame False {
                          }
                          frame True {
                            n460 = Two Button Dialog(message="Ну шо, облучаем?", 1:"Нет" ("F button name (\"Cancel\")"), 2:"Да" ("T button name (\"OK\")")) -> (T button?=w863:bool)
                          }
                        }
                      }
                      frame Enabled {
                      }
                    }
                  }
                  frame Enabled {
                    n461 = while {
                      tunnel: [w869] -> w868
                      stop <- w869 stop-if-true
                      n462 = local read "Стабилизировано"() -> (w869:bool)
                    }
                  }
                }
                "Готовы облучать" <- w855
              }
              frame #2 {
                n463 = local write "Num_hits_req"(u64 0 ("Num_hits_req")) -> ()
              }
            }
          }
        }
      }
      frame "Quit" {
        w873 = FALSE
        n464 = local write "Status:"("Выход" ("Status:")) -> ()
        n465 = local write "Num_hits"(u64 0 ("Num_hits")) -> ()
        n466 = local write "stop"(w873) -> ()
        n467 = local write "Power Enable"(w873) -> ()
        n468 = local write "Прервать"(w873) -> ()
        n469 = local write "Count_hits?"(w873) -> ()
      }
    }
  }
  n470 = while {
    tunnel: w9 -> [w878]
    stop <- FALSE stop-if-true
    n471 = event shown="[0] \"stop\": Value Change" {
      selector: _ -> [_ _ _ _]
      dyn-events: _ -> [_ _ _ _]
      timeout: _ -> [_ _ _ _]
      tunnel: w878 -> [_ _ _ _]
      event "stop": Value Change {
        # "Работает, зараза, через раз"
        n472 = event-data() -> ()  [unwired: 1 in, 6 out]
        n473 = flat-sequence {
          frame #0 {
            n474 = local write "Case"(T1."Quit" ("Case")) -> ()
          }
          frame #1 {
            n475 = local write "stop"(FALSE) -> ()
            "Прервать" <- TRUE
          }
        }
      }
      event "Раб. режим LD": Value Change {
        n476 = event-data() -> ()  [unwired: 1 in, 6 out]
        n477 = flat-sequence {
          frame #0 {
            n478 = local write "Раб. режим LD"(FALSE) -> ()
            n479 = local write "Case"(T1."Bias" ("Case")) -> ()
          }
          frame #1 {
            n480 = local write "Выполняется"(TRUE) -> ()
          }
        }
      }
      event "Хар-ка TEC": Value Change {
        n481 = event-data() -> ()  [unwired: 1 in, 6 out]
        n482 = flat-sequence {
          frame #0 {
            n483 = local write "Хар-ка TEC"(FALSE) -> ()
            n484 = local write "Case"(T1."TEC_Chars" ("Case")) -> ()
          }
          frame #1 {
            n485 = local write "Выполняется"(TRUE) -> ()
          }
        }
      }
      event "Хар-ки от I_LD": Value Change {
        n486 = event-data() -> ()  [unwired: 1 in, 6 out]
        n487 = flat-sequence {
          frame #0 {
            n488 = local write "Хар-ки от I_LD"(FALSE) -> ()
            n489 = local write "Case"(T1."Characteristics" ("Case")) -> ()
          }
          frame #1 {
            n490 = local write "Выполняется"(TRUE) -> ()
          }
        }
      }
    }
  }
  n491 = while {
    tunnel: w8 -> [w892]
    tunnel: w7 -> [w893]
    stop <- FALSE stop-if-true
    w895 = T1."Initialization"  # Case
    n492 = disable-structure shown="Enabled" {
      frame Disabled {
        n493 = local read "Выполняется"() -> (w897:bool)
        n494 = Compound Arithmetic op=OR(w897) -> ()  [unwired: 1 in, 1 out]
      }
      frame Enabled {
      }
    }
    n495 = local read "Case"() -> (w894:T1)
    n496 = Equal?(x=w894, y=w895) -> (x = y?=w891:bool)
    n497 = case shown="False" w891 {
      tunnel: w893 -> [w899 _]
      tunnel: w892 -> [w898 _]
      frame False {
        n498 = stacked-sequence {
          tunnel: w899 -> [w902 w937 _ _ _]
          tunnel: w898 -> [w901 w936 _ _ _]
          frame #0 {
            n499 = local read "Power Enable"() -> (w900:bool)
            n500 = call <instrlib>:"niDCPower Configure Output Enabled.vi"("output enabled"=w900, "channel name"="0,1,2", "instrument handle"=w902) -> ()  [unwired: 7 in, 2 out]
            n501 = call <instrlib>:"niDCPower Configure Output Enabled.vi"("output enabled"=w900, "channel name"="0,1,2", "instrument handle"=w901) -> ()  [unwired: 7 in, 2 out]
          }
          frame #1 {
            w916 = "1"
            w920 = 1000.0 ("y")
            w927 = "0" ("channel name")
            n502 = Divide(x="Предел тока ТЕС, мА", y=1000.0) -> (x/y=w930:dbl)
            n503 = call <instrlib>:"niDCPower Configure Current Limit.vi"("current limit"=w930, "channel name"="2", "instrument handle"=w937) -> ("instrument handle out"=w909:refnum<k15>)  [unwired: 7 in, 1 out]
            n504 = call <instrlib>:"niDCPower Configure Current Limit.vi"("current limit"=w930, "channel name"="0", "instrument handle"=w936) -> ("instrument handle out"=w923:refnum<k15>)  [unwired: 7 in, 1 out]
            n505 = Divide(x="Предел тока LD, мА", y=w920) -> (x/y=w931:dbl)
            n506 = Divide(x="Предел тока PDext, мА", y=w920) -> (x/y=w922:dbl)
            n507 = call <instrlib>:"niDCPower Configure Current Limit.vi"("current limit"=w922, "channel name"=w916, "instrument handle"=w923) -> ("instrument handle out"=w915:refnum<k15>)  [unwired: 7 in, 1 out]
            n508 = call <instrlib>:"niDCPower Measure Multiple.vi"("channel name"="2", "instrument handle"=w909) -> ("current measurements"=w912:dbl[])  [unwired: 6 in, 3 out]
            n509 = call <instrlib>:"niDCPower Configure Current Limit.vi"("current limit"=w931, "channel name"=w927, "instrument handle"=w909) -> ("instrument handle out"=w928:refnum<k15>)  [unwired: 7 in, 1 out]
            n510 = call <instrlib>:"niDCPower Measure Multiple.vi"("channel name"=w916, "instrument handle"=w915) -> ("current measurements"=w917:dbl[])  [unwired: 6 in, 3 out]
            n511 = Index Array(array=w912) -> (element=w911:dbl)  [unwired: 1 in]
            n512 = call <instrlib>:"niDCPower Measure Multiple.vi"("channel name"=w927, "instrument handle"=w928) -> ("current measurements"=w926:dbl[])  [unwired: 6 in, 3 out]
            n513 = Multiply(x=w911, y=1000.0) -> (x*y=w913:dbl)
            n514 = Index Array(array=w917) -> (element=w918:dbl)  [unwired: 1 in]
            n515 = Absolute Value(x=w913) -> (abs(x)=w907:dbl)
            n516 = Index Array(array=w926) -> (element=w925:dbl)  [unwired: 1 in]
            n517 = Multiply(x=w918, y=1000.0) -> (x*y=w914:dbl)
            n518 = local write "TEC_current, mA"(w907) -> ()
            n519 = Absolute Value(x=w914) -> (abs(x)=w905:dbl)
            "ExtPhotodiode Current" <- w905
            n520 = Multiply(x=w925, y=1000.0) -> (x*y=w906:dbl)
            "Operating Current" <- w906
            n521 = local write "Operating Current, mA"(w906) -> ()
            n522 = local write "IPD(ext), mA"(w905) -> ()
          }
          frame #2 {
            n523 = Wait (ms)(milliseconds to wait=u32 100) -> ()  [unwired: 1 out]
          }
          frame #3 {
            n524 = local read "Source_2_Vcc_out"() -> (w943:refnum<k15>)
            n525 = Select(t=0.0, s="Нагрев", f=-5.0) -> (s? t:f=w941:dbl)
            n526 = call <instrlib>:"niDCPower Configure Voltage Level.vi"("voltage level"=w941, "channel name"="2", "instrument handle"=w943) -> ()  [unwired: 7 in, 2 out]
          }
          frame #4 {
            w949 = T4 6.5 items=["3 1/2"=3.5, "4 1/2"=4.5, "5 1/2"=5.5, "6 1/2"=6.5, "7 1/2"=7.5] ("Resolution in Digits")
            n527 = local read "4071(1)_adress"() -> (w948:refnum<k15>)
            n528 = call-poly <instrlib>:"niDMM Config Measurement.vi"("Range"=-1.0 ("Configuration:Measurement Options:Max Frequency"), "Resolution in Digits"=w949, "Function"=niDMM_Function."DC Current" ("multimeter mode"), "instrument handle"=w948) -> ("instrument handle out"=w950:refnum<k15>)  [unwired: 6 in, 1 out]
            n529 = for {
              N: 2 -> [_]
              tunnel: w950 -> [w957]
              tunnel: [w956] -> w952 mode=indexing
              n530 = call <instrlib>:"niDMM Read.vi"("instrument handle"=w957) -> ("Measurement"=w956:dbl)  [unwired: 8 in, 2 out]
            }
            n531 = call-poly <vilib>:"Mean.vi"("X"=w952) -> ("mean"=w953:dbl)  [unwired: 1 out]
            n532 = Absolute Value(x=w953) -> (abs(x)=w954:dbl)
            n533 = Multiply(x=w954, y=1000000.0) -> (x*y=w945:dbl)
            "Monitor current, uA" <- w945
            n534 = local write "I_pd, uA"(w945) -> ()
          }
        }
      }
      frame True {
        n535 = Wait (ms)(milliseconds to wait=u32 20) -> ()  [unwired: 1 out]
      }
    }
  }
  n536 = while {
    tunnel: w7 -> [w960]
    tunnel: w8 -> [w959]
    stop <- FALSE stop-if-true
    n537 = local read "stop"() -> (w961:bool)
    n538 = case shown="True" w961 {
      tunnel: w960 -> [_ w964]
      tunnel: w959 -> [_ w963]
      frame False {
      }
      frame True {
        n539 = stacked-sequence {
          tunnel: w964 -> [_ _ _ _ w971 _]
          tunnel: w963 -> [_ _ _ _ w970 _]
          frame #0 {
            w965 = T1."Initialization"  # Case
            n540 = local write "Case"(w965) -> ()
          }
          frame #1 {
            # "Закрытие логов"
            n541 = local read "refnum out"() -> (w966:refnum<file>)
            n542 = Format Into String(initial string=w966, "\r\n") -> (resulting string=w968:refnum<file>)  [unwired: 2 in, 1 out]
            n543 = Close File(refnum=w968) -> ()  [unwired: 1 in, 2 out]
          }
          frame #2 {
            # "Выключение Офира"
          }
          frame #3 {
            w969 = FALSE
            n544 = local write "Раб. режим LD"(w969) -> ()
            n545 = local write "Хар-ки от I_LD"(w969) -> ()
            n546 = local write "Power Enable"(w969) -> ()
            n547 = local write "Хар-ка TEC"(w969) -> ()
          }
          frame #4 {
            w974 = "0,1,2" ("channel name")
            w979 = "0,1,2" ("channel name")
            n548 = call <instrlib>:"niDCPower Configure Voltage Level.vi"("voltage level"=0.0, "channel name"=w979, "instrument handle"=w971) -> ("instrument handle out"=w978:refnum<k15>)  [unwired: 7 in, 1 out]
            n549 = call <instrlib>:"niDCPower Configure Voltage Level.vi"("voltage level"=0.0, "channel name"=w974, "instrument handle"=w970) -> ("instrument handle out"=w975:refnum<k15>)  [unwired: 7 in, 1 out]
            n550 = call <instrlib>:"niDCPower Configure Output Enabled.vi"("output enabled"=FALSE, "channel name"=w979, "instrument handle"=w978) -> ("instrument handle out"=w977:refnum<k15>)  [unwired: 7 in, 1 out]
            n551 = call <instrlib>:"niDCPower Configure Output Enabled.vi"("output enabled"=FALSE, "channel name"=w974, "instrument handle"=w975) -> ("instrument handle out"=w976:refnum<k15>)  [unwired: 7 in, 1 out]
            n552 = call <instrlib>:"niDCPower Close.vi"("instrument handle"=w977) -> ()  [unwired: 10 in, 1 out]
            n553 = call <instrlib>:"niDCPower Close.vi"("instrument handle"=w976) -> ()  [unwired: 10 in, 1 out]
          }
          frame #5 {
            n554 = Stop(stop? (T)=TRUE) -> ()
          }
        }
      }
    }
  }
  n555 = disable-structure shown="Disabled" {
    frame Disabled {
      n556 = local read "4070_address"() -> (w986:refnum<k15>)
      n557 = local read "TEC_Source"() -> (w983:enum16{"S1_Ch2", "S2_Ch0", "S3_Ch1"})
      n558 = case shown="\"S3_Ch1\"" w983 {
        tunnel: [w996 w998 w1000] -> w985
        tunnel: ["2" "0" "1"] -> w984
        frame "S1_Ch2", Default {
          n559 = local read "Source_1_Vcc_out"() -> (w996:refnum<k15>)
        }
        frame "S2_Ch0" {
          n560 = local read "Source_2_Vcc_out"() -> (w998:refnum<k15>)
        }
        frame "S3_Ch1" {
          n561 = local read "Source_3_Vcc_out"() -> (w1000:refnum<k15>)
        }
      }
      n562 = call "Res_stabiliz.vi"("Точность ThRes"="Точность ThRes", "Up_Volt_limit"="the upper limit for the voltage", "Optimum ThRes"="Optimum ThRes", "Low_Volt_limit"="the lower limit for the voltage", "TEC_Source"=w985, "4070_address"=w986, "channel name"=w984) -> ("Подстроенное напряжение"=→"Подстроенное напряжение\nстабилизации":dbl, "ThRes value"=→"ThRes value":dbl, "thRes_adj"=w994:dbl, "Start Voltage"=w987:dbl)  [unwired: 1 out]
      n563 = local write "Сопротивление терморез-ра"(w994) -> ()
    }
    frame Enabled {
    }
  }
  n564 = disable-structure shown="Disabled" {
    frame Disabled {
      w1006 = T4 6.5 items=["3 1/2"=3.5, "4 1/2"=4.5, "5 1/2"=5.5, "6 1/2"=6.5, "7 1/2"=7.5] ("Resolution in Digits")
      n565 = local read "4070_address"() -> (w1005:refnum<k15>)
      n566 = call-poly <instrlib>:"niDMM Config Measurement.vi"("Range"=-1.0 ("Configuration:Measurement Options:Max Frequency"), "Resolution in Digits"=w1006, "Function"=niDMM_Function."2-wire Resistance" ("multimeter mode"), "instrument handle"=w1005) -> ("instrument handle out"=w1004:refnum<k15>)  [unwired: 6 in, 1 out]
      n567 = for {
        N: 3 -> [_]
        tunnel: w1004 -> [w1010]
        tunnel: [w1009] -> w1003 mode=indexing
        n568 = call <instrlib>:"niDMM Read.vi"("instrument handle"=w1010) -> ("Measurement"=w1009:dbl)  [unwired: 8 in, 2 out]
        n569 = Wait (ms)(milliseconds to wait=u32 50) -> ()  [unwired: 1 out]
      }
      n570 = call-poly <vilib>:"Mean.vi"("X"=w1003) -> ("mean"=→"Сопротивление терморез-ра":dbl)  [unwired: 1 out]
    }
    frame Enabled {
    }
  }
  n571 = local write "Нагрев"(FALSE ("Нагрев")) -> ()
  n572 = disable-structure shown="Enabled" {
    frame Disabled {
      # "Есть в инициализации"
      # "Для измерения Сопротивления"
      # "Поменять in0/in1 для ТЕС"
      n573 = local read "Source_2_Vcc_out"() -> (w1017:refnum<k15>)
      n574 = local read "4070_Rele_source"() -> (w1012:enum16{"S2_Ch0", "S1_Ch2"})
      n575 = call <instrlib>:"niDCPower Configure Voltage Level.vi"("voltage level"=-5.0, "channel name"="2", "instrument handle"=w1017) -> ()  [unwired: 7 in, 2 out]
      n576 = case shown="\"S1_Ch2\"" w1012 {
        tunnel: [5.0 -5.0] -> w1013
        tunnel: ["0" "2"] -> w1014
        tunnel: [w1019 w1022] -> w1015
        frame "S2_Ch0", Default {
          n577 = local read "Source_2_Vcc_out"() -> (w1019:refnum<k15>)
        }
        frame "S1_Ch2" {
          n578 = local read "Source_1_Vcc_out"() -> (w1022:refnum<k15>)
        }
      }
      n579 = call <instrlib>:"niDCPower Configure Voltage Level.vi"("voltage level"=w1013, "channel name"=w1014, "instrument handle"=w1015) -> ()  [unwired: 7 in, 2 out]
    }
    frame Enabled {
    }
  }
  "Выполняется" <- w4
